vi "SCA-RT.vi"() -> ()   [LabVIEW 2016]
uses:
  Controls/SCA states.ctl
  Controls/Gate Valve Readback.ctl
  Controls/Vertical Rod states.ctl
  Controls/Horizontal Rod states.ctl
  Controls/GP307 cluster.ctl
  Controls/SCA commands.ctl
  Controls/SCA Bypass control.ctl
  Controls/Sample Changer Settings.ctl
  <vilib>/Platform/TimedLoop/XDataNode/timing_clust.ctl
  <vilib>/Platform/TimedLoop/XDataNode/nitl_modes.ctl
  <vilib>/Platform/TimedLoop/XDataNode/wakeup.ctl
  Controls/Encoder bit cluster.ctl
  Controls/Minimum Times.ctl
  <vilib>/Analysis/baseanly.llb/Mean (DBL).vi
  <vilib>/Instr/_visa.llb/VISA Configure Serial Port (Instr).vi
  <vilib>/Motion/Express/_s/nimc.fb.straightLineMove.startStraightLineMove.axis.modeRelative.0.vi
  <vilib>/Platform/TimedLoop/XDataNode/loadnilvce.vi
  <vilib>/Motion/BlockNode/FB.NIMotion.xnode
  <vilib>/Platform/TimedLoop/XDataNode/XDataNode.xnode
  <vilib>/Platform/TimedLoop/XDataNode/XDNodeRunTimeDep.lvlib
  <vilib>/Analysis/NI_AALBase.lvlib
  <vilib>/NI_Real-Time Target Support.lvlib
panel:
  out "Encoder Offset":i32
  out "SCA settings":T1
  out "Bypass error":errorcluster
  out "HV Readback error":errorcluster
  out "SCA command monitor error":errorcluster
  in  "Insert Rod Bypass":bool
  in  "Retract Rod Bypass":bool
  in  "Sample Rod Bypass":bool
  in  "Wheel GV Bypass":bool
  out "Bypass Control":T2
  out "Timeouts":T3
  out "Immersion Lens I set":dbl
  out "Immersion Lens V Set":dbl
  out "Settings Update error":errorcluster
  out "SCA Command":T4=enum."Retract insert rod"
  out "Encoder error":errorcluster
  out "Convectron readback error":errorcluster
  out "HV Control error":errorcluster
  out "Rotate Wheel error":errorcluster
  out "Ion Source Vac Cluster":T5
  out "Bellows Vac Cluster":T5
  out "SCA-cRIO error":errorcluster
  out "Rollover Sample":u16=54
  out "Insert Rod Status":T6
  out "Retract Rod Status":T6
  out "Sample Rod status":T7
  out "Wheel GV":T8
  out "Raw bits":bool[](array[boolean])
  out "Converted bits":bool[](array[boolean])
  out "Immersion Lens I read":dbl format="%0.2f"
  out "Immersion Lens V read":dbl format="%0.2f"
  out "SCA next state":T9
  out "Extractor I read":dbl
  out "Extractor V read":dbl
  out "Extractor V set":dbl
  out "Cathode V read":dbl
  out "Cathode I read":dbl
  out "Cathode V set":dbl
  out "New Move":dbl
  out "Encoder Destination":dbl
  out "Step Window Radius":u8=2
  out "In Range?":bool
  out "Window Limit 2":u32
  out "Window Limit 1":u32
  out "Encoder position":u16
  out "action":string
  out "Vac Readback error":errorcluster
  out "Sample Wheel Convectron":string
  out "Sample Rod UP sensor":bool
  out "Sample Rod DOWN sensor":bool
  out "Rotation done":bool
  out "Insert Rod IN sensor":bool
  out "Insert Rod OUT sensor":bool
  out "Retract Rod IN sensor":bool
  out "Retract Rod OUT sensor":bool
  out "Sensor error":errorcluster
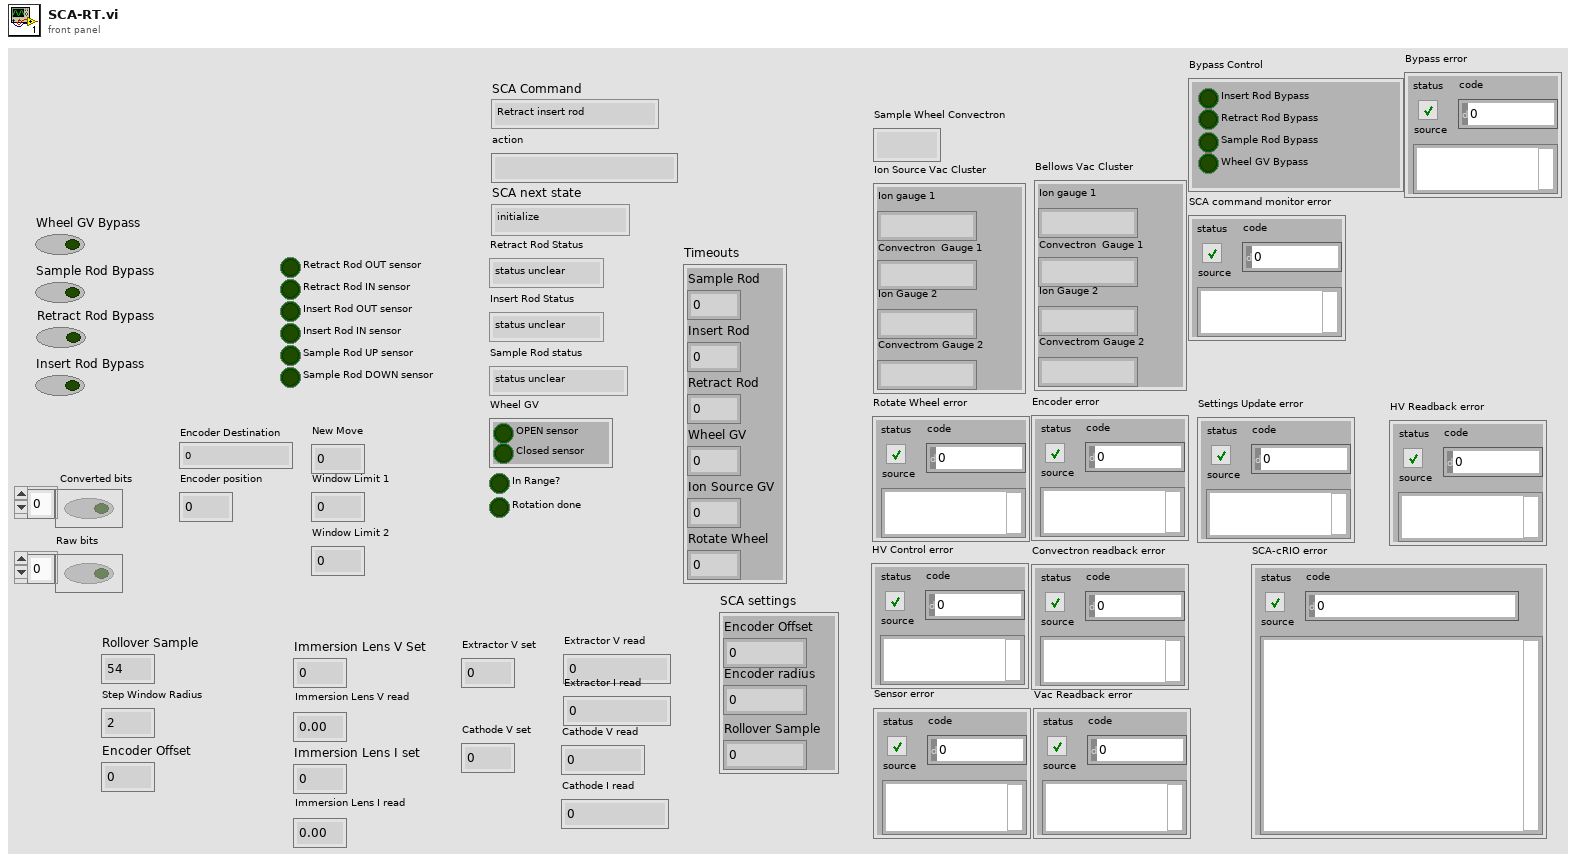
[diagram p1: front panel]
types:
  T1 = typedef "Sample Changer Settings.ctl" = cluster{"Encoder Offset":i32, "Encoder radius":u8, "Rollover Sample":u16}
  T2 = typedef "SCA Bypass control.ctl" = cluster{"Insert Rod Bypass":bool, "Retract Rod Bypass":bool, "Sample Rod Bypass":bool, "Wheel GV Bypass":bool}
  T3 = cluster{"Sample Rod":u16, "Insert Rod":u16, "Retract Rod":u16, "Wheel GV":u16, "Ion Source GV":u16, "Rotate Wheel":u16}
  T4 = typedef "SCA commands.ctl" = enum16{"Wait", "Shutdown", "Retract insert rod", "Insert insert rod", "Retract retract rod", "Insert retract rod", "Retract sample rod", "Insert sample rod", "Open wheel GV", "Close wheel GV", "Open ion source GV", "Close ion source GV", "Pump out source", "Vent source", "Rotate wheel randomly", "Rotate wheel", "Start random sample change", "Start sample change"}
  T5 = typedef "GP307 cluster.ctl" = cluster{"Ion gauge 1":string, "Convectron  Gauge 1 ":string, "Ion Gauge 2":string, "Convectrom Gauge 2":string}
  T6 = typedef "Horizontal Rod states.ctl" = enum16{"status unclear", "rod in", "rod out"}
  T7 = typedef "Vertical Rod states.ctl" = enum16{"status unclear", "rod down", "rod up"}
  T8 = typedef "Gate Valve Readback.ctl" = cluster{"OPEN sensor":bool, "Closed sensor":bool}
  T9 = typedef "SCA states.ctl" = enum16{"initialize", "wait", "change sample start", "change sample", "check position", "rotate wheel", "sample change complete", "sample rod up", "sample rod down", "retract rod in", "retract rod out", "insert rod in", "insert rod out", "wheel GV open", "wheel GV close", "vent source", "pump source", "shutdown"}
  T10 = cluster{"Sample Rod":u32, "Insert Rod":u32, "Retract Rod":u32, "Wheel GV":u32, "Ion Source GV":u32, "Rotate Wheel":u32}
  T11 = typedef "Minimum Times.ctl" = cluster{"Rotate Wheel Minimum Time":u32}
  T12 = typedef "XDNodeRunTimeDep.lvlib/timing_clust.ctl" = cluster{"Expected End [f-1]":u64, "Actual End [f-1]":u64, "Finished Late? [f-1]":bool, "Expected End [i-1]":u64, "Actual End [i-1]":u64, "Finished Late? [i-1]":bool, "Expected Start [i]":u64, "Actual Start [i]":u64, "Expected Start [f]":u64, "Actual Start [f]":u64, "Source Name":string, "Structure Name":string, "Period":i64, "Deadline":i64, "Offset":i64, "Start":i64, "Priority":i32, "Timeout":i32, "Mode":T13, "Wakeup Reason":T14, "Error":errorcluster, "Source Type":string, "Secondary Source Type":string, "Global End Time":u64, "Global Start Time":u64, "Frame Duration":u64, "Iteration Duration":u64, "Assigned CPU":i32, "I/O Scan Engine Mode":u32}
  T13 = typedef "XDNodeRunTimeDep.lvlib/nitl_modes.ctl" = enum32{"No Change", "Process missed periods, maintain original phase", "Discard missed periods, maintain original phase", "Process missed periods, ignore original phase", "Discard missed periods, ignore original phase"}
  T14 = typedef "XDNodeRunTimeDep.lvlib/wakeup.ctl" = enum32{"Normal", "Aborted", "Asynchronous wakeup", "Timing source error", "Timed loop error", "Timeout"}
  T15 = typedef "Encoder bit cluster.ctl" = cluster{"MSB":bool, "13th bit":bool, "12th bit":bool, "11th bit":bool, "10th bit":bool, "9th bit":bool, "8th bit":bool, "7th bit":bool, "6th bit":bool, "5th bit":bool, "4th bit":bool, "3rd bit":bool, "2nd bit":bool, "LSB":bool}
  T16 = typedef "GV states.ctl" = enum16{"status unclear", "closed", "open"}
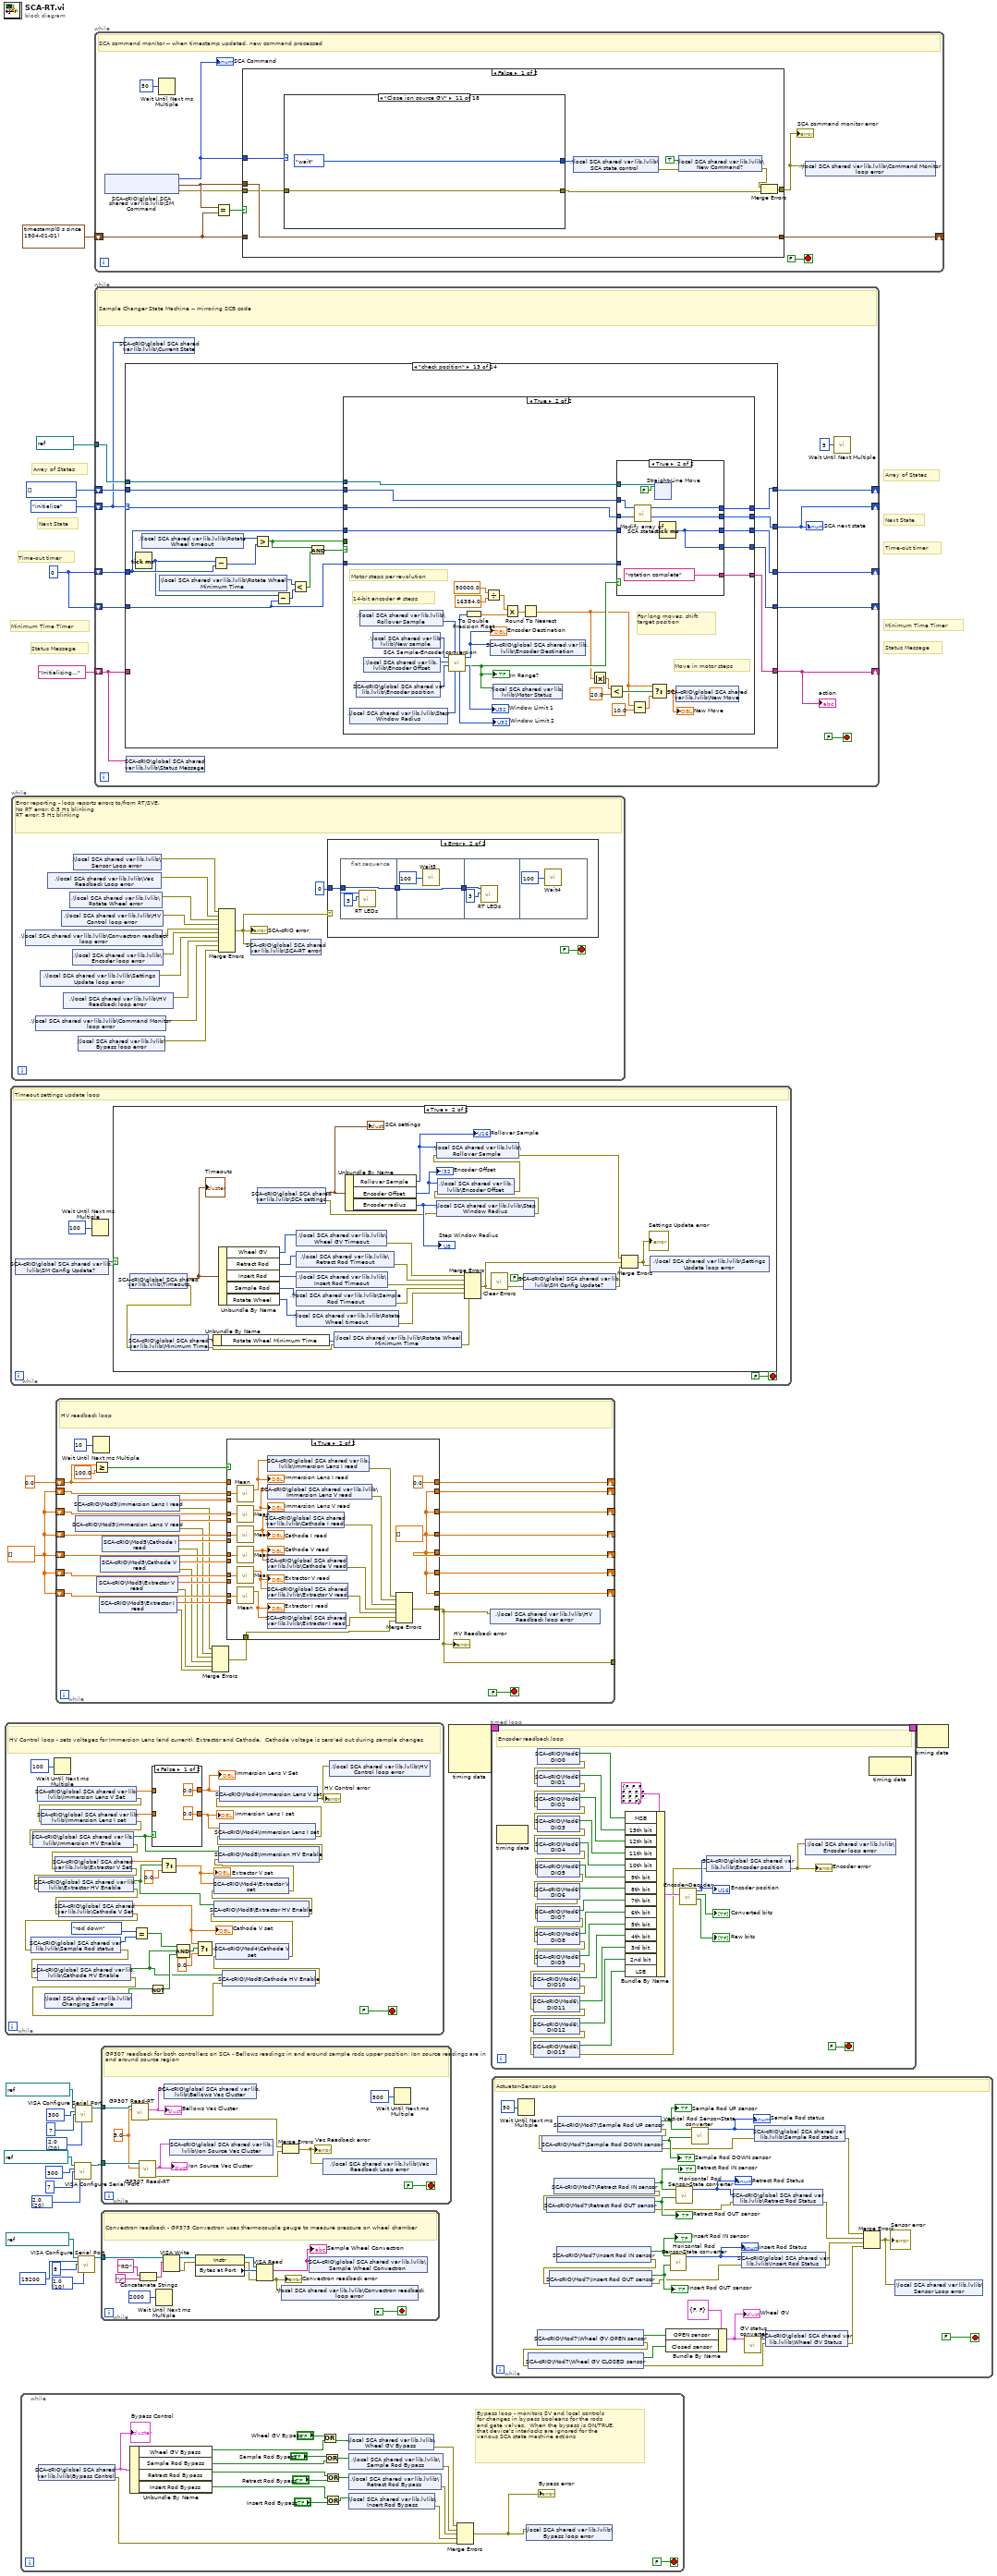
[diagram p0: block diagram]
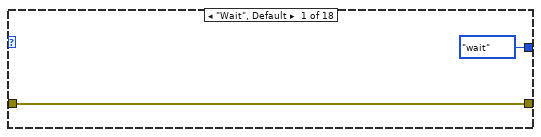
[diagram p2: hidden frame]
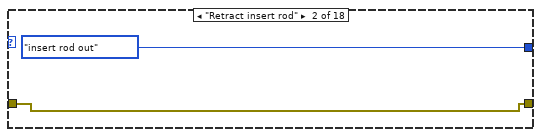
[diagram p3: hidden frame]
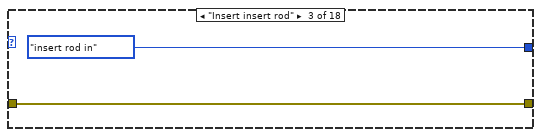
[diagram p4: hidden frame]
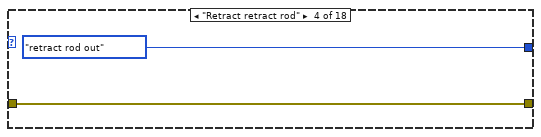
[diagram p5: hidden frame]
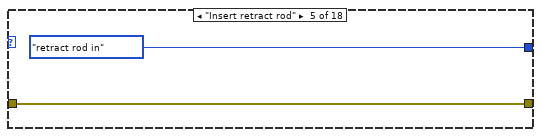
[diagram p6: hidden frame]
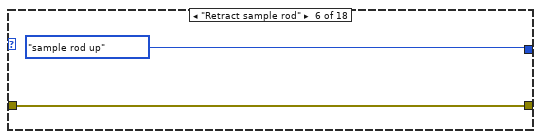
[diagram p7: hidden frame]
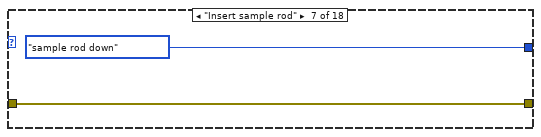
[diagram p8: hidden frame]
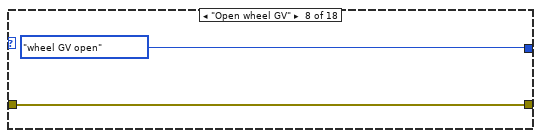
[diagram p9: hidden frame]
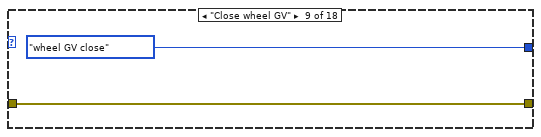
[diagram p10: hidden frame]
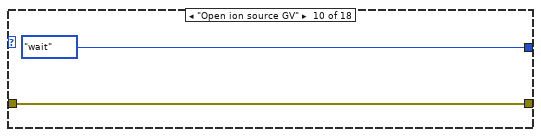
[diagram p11: hidden frame]
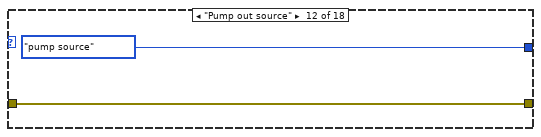
[diagram p12: hidden frame]
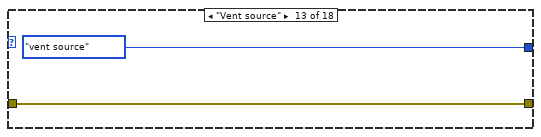
[diagram p13: hidden frame]
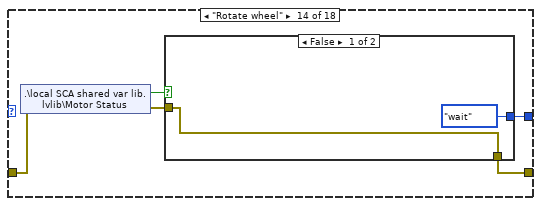
[diagram p14: hidden frame]
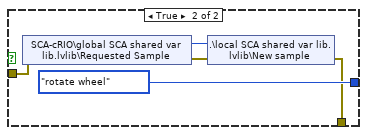
[diagram p15: hidden frame]
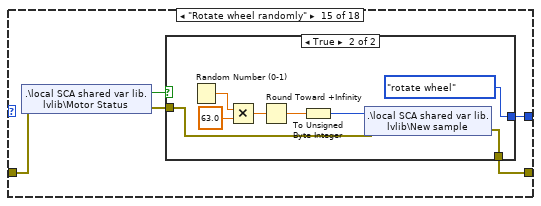
[diagram p16: hidden frame]
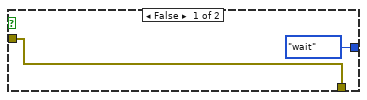
[diagram p17: hidden frame]
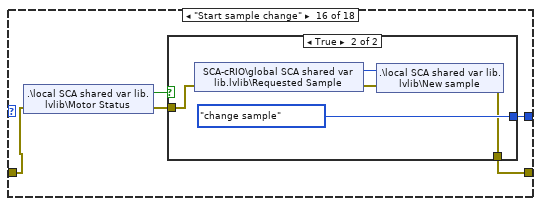
[diagram p18: hidden frame]
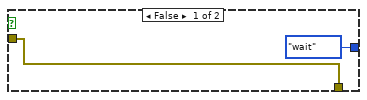
[diagram p19: hidden frame]
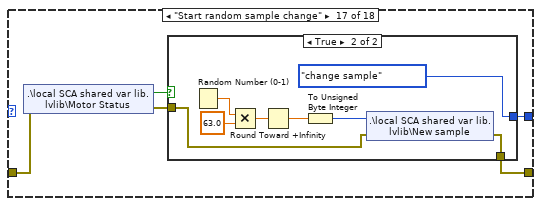
[diagram p20: hidden frame]
diagram:
  w3 = dbl[] []
  w20 = u16 20 items=["1.0"=10, "1.5"=15, "2.0"=20] ("stop bits (10: 1 bit)")
  w24 = u16 10 items=["1.0"=10, "1.5"=15, "2.0"=20] ("stop bits (10: 1 bit)")
  w14 = u16 20 items=["1.0"=10, "1.5"=15, "2.0"=20] ("stop bits (10: 1 bit)")
  w8 = u32 0
  w25 = T9[] [] items=["initialize", "wait", "change sample start", "change sample", "check position", "rotate wheel", "sample change complete", "sample rod up", "sample rod down", "retract rod in", "retract rod out", "insert rod in", "insert rod out", "wheel GV open", "wheel GV close", "vent source", "pump source", "shutdown"]
  # "Status Message"
  # "Array of States"
  # "Next State"
  # "Time-out timer"
  # "Minimum Time Timer"
  # "Status Message"
  # "Array of States"
  # "Next State"
  # "Time-out timer"
  # "Minimum Time Timer"
  n1 = while {
    stop <- FALSE stop-if-true
    # "HV Control loop - sets voltages for Immersion Lens (and current), Extractor and Cathode.  Cathode voltage is zero'ed out during sample changes"
    n2 = shared-variable "SCA-cRIO\\global SCA shared var lib.lvlib\\Immersion Lens V Set"() -> (w47:dbl, error out=w54:errorcluster)  [unwired: 1 in]
    n3 = shared-variable "SCA-cRIO\\global SCA shared var lib.lvlib\\Immersion Lens I set"(error in=w54) -> (w45:dbl, error out=w43:errorcluster)
    n4 = shared-variable "SCA-cRIO\\global SCA shared var lib.lvlib\\Immersion HV Enable"(error in=w43) -> (w27:bool, error out=w42:errorcluster)
    n5 = shared-variable ".\\local SCA shared var lib.lvlib\\Changing Sample"() -> (w59:bool)  [unwired: 1 in, 1 out]
    n6 = Wait Until Next ms Multiple(millisecond multiple=u32 100) -> ()  [unwired: 1 out]
    n7 = shared-variable "SCA-cRIO\\global SCA shared var lib.lvlib\\Extractor V Set"(error in=w42) -> (w40:dbl, error out=w41:errorcluster)
    n8 = shared-variable "SCA-cRIO\\global SCA shared var lib.lvlib\\Extractor HV Enable"(error in=w41) -> (w26:bool, error out=w37:errorcluster)
    n9 = shared-variable "SCA-cRIO\\global SCA shared var lib.lvlib\\Cathode V Set"(error in=w37) -> (w57:dbl, error out=w53:errorcluster)
    "Cathode V set" <- w57
    n10 = shared-variable "SCA-cRIO\\global SCA shared var lib.lvlib\\Sample Rod status"(error in=w53) -> (w49:T7, error out=w35:errorcluster)
    n11 = shared-variable "SCA-cRIO\\global SCA shared var lib.lvlib\\Cathode HV Enable"(error in=w35) -> (w34:bool, error out=w33:errorcluster)
    n12 = Equal?(x=Vertical_Rod_states."rod down", y=w49) -> (x = y?=w50:bool)
    n13 = Not(x=w59) -> (.not. x?=w36:bool)
    n14 = case shown="False" w27 {
      tunnel: [0.0 ("Double") w65] -> w46
      tunnel: w47 -> [_ w65]
      tunnel: w45 -> [_ w64]
      tunnel: [0.0 ("Double") w64] -> w44
      frame False {
      }
      frame True {
      }
    }
    "Immersion Lens V Set" <- w46
    "Immersion Lens I set" <- w44
    n15 = Select(t=w40, s=w26, f=0.0) -> (s? t:f=w39:dbl)
    "Extractor V set" <- w39
    n16 = Compound Arithmetic op=AND(w50, w34, w36) -> (w58:bool)
    n17 = Select(t=w57, s=w58, f=0.0) -> (s? t:f=w55:dbl)
    n18 = shared-variable "SCA-cRIO\\Mod8\\Cathode HV Enable"(w34, error in=w33) -> (error out=w32:errorcluster)
    n19 = shared-variable "SCA-cRIO\\Mod4\\Cathode V set"(w55, error in=w32) -> (error out=w31:errorcluster)
    n20 = shared-variable "SCA-cRIO\\Mod8\\Extractor HV Enable"(w26, error in=w31) -> (error out=w30:errorcluster)
    n21 = shared-variable "SCA-cRIO\\Mod4\\Extractor V set"(w39, error in=w30) -> (error out=w28:errorcluster)
    n22 = shared-variable "SCA-cRIO\\Mod8\\Immersion HV Enable"(w27, error in=w28) -> (error out=w29:errorcluster)
    n23 = shared-variable "SCA-cRIO\\Mod4\\Immersion Lens I set"(w44, error in=w29) -> (error out=w52:errorcluster)
    n24 = shared-variable "SCA-cRIO\\Mod4\\Immersion Lens V set"(w46, error in=w52) -> (error out=w51:errorcluster)
    "HV Control error" <- w51
    n25 = shared-variable ".\\local SCA shared var lib.lvlib\\HV Control loop error"(w51) -> ()  [unwired: 1 in, 1 out]
  }
  n26 = while {
    stop <- FALSE stop-if-true
    # "Timeout settings update loop"
    n27 = shared-variable "SCA-cRIO\\global SCA shared var lib.lvlib\\SM Config Update?"() -> (w68:bool)  [unwired: 1 in, 1 out]
    n28 = Wait Until Next ms Multiple(millisecond multiple=u32 100) -> ()  [unwired: 1 out]
    n29 = case shown="True" w68 {
      frame False {
      }
      frame True {
        n30 = shared-variable "SCA-cRIO\\global SCA shared var lib.lvlib\\Timeouts"() -> (w96:T10, error out=w79:errorcluster)  [unwired: 1 in]
        "Timeouts" <- w96
        n31 = shared-variable "SCA-cRIO\\global SCA shared var lib.lvlib\\Minimum Time"(error in=w79) -> (w81:T11, error out=w78:errorcluster)
        n32 = Unbundle By Name(w81) -> ("Rotate Wheel Minimum Time"=w80:u32)
        n33 = Unbundle By Name(w96) -> ("Wheel GV"=w95:u32, "Retract Rod"=w82:u32, "Insert Rod"=w89:u32, "Sample Rod"=w86:u32, "Rotate Wheel"=w85:u32)
        n34 = shared-variable "SCA-cRIO\\global SCA shared var lib.lvlib\\SCA settings"() -> (w76:T1, error out=w73:errorcluster)  [unwired: 1 in]
        "SCA settings" <- w76
        n35 = shared-variable ".\\local SCA shared var lib.lvlib\\Wheel GV Timeout"(w95) -> (error out=w94:errorcluster)  [unwired: 1 in]
        n36 = shared-variable ".\\local SCA shared var lib.lvlib\\Retract Rod Timeout"(w82) -> (error out=w88:errorcluster)  [unwired: 1 in]
        n37 = shared-variable ".\\local SCA shared var lib.lvlib\\Insert Rod Timeout"(w89) -> (error out=w87:errorcluster)  [unwired: 1 in]
        n38 = shared-variable ".\\local SCA shared var lib.lvlib\\Sample Rod Timeout"(w86) -> (error out=w84:errorcluster)  [unwired: 1 in]
        n39 = shared-variable ".\\local SCA shared var lib.lvlib\\Rotate Wheel timeout"(w85) -> (error out=w83:errorcluster)  [unwired: 1 in]
        n40 = shared-variable ".\\local SCA shared var lib.lvlib\\Rotate Wheel Minimum Time"(w80, error in=w78) -> (error out=w77:errorcluster)
        n41 = Unbundle By Name(w76) -> ("Rollover Sample"=w71:u16, "Encoder Offset"=w74:i32, "Encoder radius"=w75:u8)
        "Step Window Radius" <- w75
        "Rollover Sample" <- w71
        "Encoder Offset" <- w74
        n42 = shared-variable ".\\local SCA shared var lib.lvlib\\Step Window Radius"(w75, error in=w73) -> (error out=w72:errorcluster)
        n43 = shared-variable ".\\local SCA shared var lib.lvlib\\Encoder Offset"(w74, error in=w72) -> (error out=w70:errorcluster)
        n44 = shared-variable ".\\local SCA shared var lib.lvlib\\Rollover Sample"(w71, error in=w70) -> (error out=w69:errorcluster)
        n45 = Merge Errors(w94, w88, w87, w84, w83, w77) -> (w92:errorcluster)
        n46 = call <vilib>:"Clear Errors.vi"("error in (no error)"=w92) -> ("error out"=w93:errorcluster)  [unwired: 5 in, 1 out]
        n47 = shared-variable "SCA-cRIO\\global SCA shared var lib.lvlib\\SM Config Update?"(FALSE ("SM Config Update?"), error in=w93) -> (error out=w91:errorcluster)
        n48 = Merge Errors(w69, w92, w91) -> (w90:errorcluster)
        "Settings Update error" <- w90
        n49 = shared-variable ".\\local SCA shared var lib.lvlib\\Settings Update loop error"(w90) -> ()  [unwired: 1 in, 1 out]
      }
    }
  }
  n50 = while {
    stop <- FALSE stop-if-true
    # "Error reporting - loop reports errors to/from RT/SVE. \nNo RT error: 0.5 Hz blinking\nRT error: 5 Hz blinking"
    n51 = shared-variable ".\\local SCA shared var lib.lvlib\\Convectron readback loop error"() -> (w103:errorcluster)  [unwired: 1 in, 1 out]
    n52 = shared-variable ".\\local SCA shared var lib.lvlib\\Command Monitor loop error"() -> (w99:errorcluster)  [unwired: 1 in, 1 out]
    n53 = shared-variable ".\\local SCA shared var lib.lvlib\\Settings Update loop error"() -> (w101:errorcluster)  [unwired: 1 in, 1 out]
    n54 = shared-variable ".\\local SCA shared var lib.lvlib\\Vac Readback Loop error"() -> (w108:errorcluster)  [unwired: 1 in, 1 out]
    n55 = shared-variable ".\\local SCA shared var lib.lvlib\\HV Control loop error"() -> (w104:errorcluster)  [unwired: 1 in, 1 out]
    n56 = shared-variable ".\\local SCA shared var lib.lvlib\\HV Readback loop error"() -> (w100:errorcluster)  [unwired: 1 in, 1 out]
    n57 = shared-variable ".\\local SCA shared var lib.lvlib\\Rotate Wheel error"() -> (w105:errorcluster)  [unwired: 1 in, 1 out]
    n58 = shared-variable ".\\local SCA shared var lib.lvlib\\Encoder loop error"() -> (w102:errorcluster)  [unwired: 1 in, 1 out]
    n59 = shared-variable ".\\local SCA shared var lib.lvlib\\Sensor Loop error"() -> (w109:errorcluster)  [unwired: 1 in, 1 out]
    n60 = shared-variable ".\\local SCA shared var lib.lvlib\\Bypass loop error"() -> (w98:errorcluster)  [unwired: 1 in, 1 out]
    n61 = Merge Errors(w109, w108, w105, w104, w103, w102, w101, w100, w99, w98) -> (w107:errorcluster)
    "SCA-cRIO error" <- w107
    n62 = shared-variable "SCA-cRIO\\global SCA shared var lib.lvlib\\SCA-RT error"(w107) -> ()  [unwired: 1 in, 1 out]
    n63 = case shown="Error" w107 {
      tunnel: 0 -> [w113 w121]
      frame No Error {
        n64 = flat-sequence {
          tunnel: w113 -> [w114]
          tunnel: [w114] -> w111
          tunnel: [w116] -> w112
          tunnel: w111 -> [w116]
          tunnel: w112 -> [w118]
          frame #0 {
            n65 = call <vilib>:"RT LEDs.vi"("State"=3, "LED Num"=w114) -> ()  [unwired: 4 in, 2 out]
          }
          frame #1 {
            n66 = call "Wait"("Count(mSec)"=u16 1000) -> ()  [unwired: 1 out]
          }
          frame #2 {
            n67 = call <vilib>:"RT LEDs.vi"("State"=3, "LED Num"=w118) -> ()  [unwired: 4 in, 2 out]
          }
          frame #3 {
            n68 = call "Wait2"("Count(mSec)"=u16 1000) -> ()  [unwired: 1 out]
          }
        }
      }
      frame Error {
        n69 = flat-sequence {
          tunnel: [w124] -> w123
          tunnel: w121 -> [w124]
          tunnel: w123 -> [w126]
          tunnel: [w126] -> w122
          tunnel: w122 -> [w128]
          frame #0 {
            n70 = call <vilib>:"RT LEDs.vi"("State"=3, "LED Num"=w124) -> ()  [unwired: 4 in, 2 out]
          }
          frame #1 {
            n71 = call "Wait3"("Count(mSec)"=u16 100) -> ()  [unwired: 1 out]
          }
          frame #2 {
            n72 = call <vilib>:"RT LEDs.vi"("State"=3, "LED Num"=w128) -> ()  [unwired: 4 in, 2 out]
          }
          frame #3 {
            n73 = call "Wait4"("Count(mSec)"=u16 100) -> ()  [unwired: 1 out]
          }
        }
      }
    }
  }
  n74 = while {
    stop <- FALSE stop-if-true
    # "Bypass loop - monitors SV and local controls\nfor changes in bypass booleans for the rods \nand gate valves.  When the bypass is ON/TRUE,\nthat device's interlocks are ignored for the \nvarious SCA state machine actions"
    n75 = shared-variable "SCA-cRIO\\global SCA shared var lib.lvlib\\Bypass Control"() -> (w144:T2, error out=w132:errorcluster)  [unwired: 1 in]
    "Bypass Control" <- w144
    n76 = Unbundle By Name(w144) -> ("Wheel GV Bypass"=w141:bool, "Sample Rod Bypass"=w140:bool, "Retract Rod Bypass"=w139:bool, "Insert Rod Bypass"=w138:bool)
    n77 = Or(x="Wheel GV Bypass", y=w141) -> (x .or. y?=w148:bool)
    n78 = Or(x="Sample Rod Bypass", y=w140) -> (x .or. y?=w147:bool)
    n79 = Or(x=w139, y="Retract Rod Bypass") -> (x .or. y?=w145:bool)
    n80 = Or(x=w138, y="Insert Rod Bypass") -> (x .or. y?=w146:bool)
    n81 = shared-variable ".\\local SCA shared var lib.lvlib\\Wheel GV Bypass"(w148) -> (error out=w136:errorcluster)  [unwired: 1 in]
    n82 = shared-variable ".\\local SCA shared var lib.lvlib\\Sample Rod Bypass"(w147) -> (error out=w135:errorcluster)  [unwired: 1 in]
    n83 = shared-variable ".\\local SCA shared var lib.lvlib\\Retract Rod Bypass"(w145) -> (error out=w134:errorcluster)  [unwired: 1 in]
    n84 = shared-variable ".\\local SCA shared var lib.lvlib\\Insert Rod Bypass"(w146) -> (error out=w133:errorcluster)  [unwired: 1 in]
    n85 = Merge Errors(w136, w135, w134, w133, w132) -> (w131:errorcluster)
    "Bypass error" <- w131
    n86 = shared-variable ".\\local SCA shared var lib.lvlib\\Bypass loop error"(w131) -> ()  [unwired: 1 in, 1 out]
  }
  n87 = while {
    shift-right: [w175] -> _
    shift-left: 0.0 ("AI1") -> [w178]
    shift-right: [w173] -> _
    shift-left: w3 -> [w172]
    shift-right: [w174] -> _
    shift-left: w3 -> [w171]
    shift-right: [w169] -> _
    shift-left: w3 -> [w168]
    shift-right: [w166] -> _
    shift-left: w3 -> [w165]
    shift-right: [w160] -> _
    shift-left: w3 -> [w163]
    shift-right: [w159] -> _
    shift-left: w3 -> [w164]
    tunnel: [w151] -> _
    stop <- FALSE stop-if-true
    # "HV readback loop"
    n88 = shared-variable "SCA-cRIO\\Mod5\\Immersion Lens V read"() -> (w161:dbl, error out=w157:errorcluster)  [unwired: 1 in]
    n89 = shared-variable "SCA-cRIO\\Mod5\\Immersion Lens I read"() -> (w162:dbl, error out=w158:errorcluster)  [unwired: 1 in]
    n90 = Wait Until Next ms Multiple(millisecond multiple=u32 10) -> ()  [unwired: 1 out]
    n91 = Greater Or Equal?(x=w178, y=100.0) -> (x >= y?=w176:bool)
    n92 = shared-variable "SCA-cRIO\\Mod5\\Extractor V read"() -> (w170:dbl, error out=w154:errorcluster)  [unwired: 1 in]
    n93 = shared-variable "SCA-cRIO\\Mod5\\Extractor I read"() -> (w167:dbl, error out=w153:errorcluster)  [unwired: 1 in]
    n94 = shared-variable "SCA-cRIO\\Mod5\\Cathode V read"() -> (w180:dbl, error out=w155:errorcluster)  [unwired: 1 in]
    n95 = shared-variable "SCA-cRIO\\Mod5\\Cathode I read"() -> (w179:dbl, error out=w156:errorcluster)  [unwired: 1 in]
    n96 = Merge Errors(w158, w157, w156, w155, w154, w153) -> (w152:errorcluster)
    n97 = case shown="True" w176 {
      tunnel: w180 -> [w199 _]
      tunnel: w179 -> [w200 _]
      tunnel: w178 -> [w203 _]
      tunnel: [w202 0.0 ("AI1")] -> w175
      tunnel: [w201 w215] -> w174
      tunnel: [w198 w215] -> w173
      tunnel: w172 -> [w197 w223]
      tunnel: w171 -> [w196 w224]
      tunnel: w170 -> [w195 _]
      tunnel: [w194 w215] -> w169
      tunnel: w168 -> [w193 w222]
      tunnel: w167 -> [w192 _]
      tunnel: [w191 w215] -> w166
      tunnel: w165 -> [w190 w221]
      tunnel: w164 -> [w189 w214]
      tunnel: w163 -> [w188 w213]
      tunnel: w162 -> [w187 _]
      tunnel: w161 -> [w186 _]
      tunnel: [w185 w215] -> w160
      tunnel: [w184 w215] -> w159
      tunnel: w152 -> [w183 w210]
      tunnel: [w183 w204] -> w151
      frame False {
        n98 = Build Array (concatenate)(w187, w188) -> (w185:dbl[])
        n99 = Build Array (concatenate)(w186, w189) -> (w184:dbl[])
        n100 = Build Array (concatenate)(w200, w196) -> (w201:dbl[])
        n101 = Build Array (concatenate)(w199, w197) -> (w198:dbl[])
        n102 = Build Array (concatenate)(w195, w193) -> (w194:dbl[])
        n103 = Build Array (concatenate)(w192, w190) -> (w191:dbl[])
        n104 = Increment(x=w203) -> (x+1=w202:dbl)
      }
      frame True {
        w215 = dbl[] []
        n105 = call-poly <vilib>:"Mean.vi"("X"=w213) -> ("mean"=w212:dbl)  [unwired: 1 out]
        "Immersion Lens I read" <- w212
        n106 = call-poly <vilib>:"Mean.vi"("X"=w214) -> ("mean"=w216:dbl)  [unwired: 1 out]
        "Immersion Lens V read" <- w216
        n107 = call-poly <vilib>:"Mean.vi"("X"=w224) -> ("mean"=w220:dbl)  [unwired: 1 out]
        "Cathode I read" <- w220
        n108 = call-poly <vilib>:"Mean.vi"("X"=w223) -> ("mean"=w219:dbl)  [unwired: 1 out]
        "Cathode V read" <- w219
        n109 = call-poly <vilib>:"Mean.vi"("X"=w222) -> ("mean"=w218:dbl)  [unwired: 1 out]
        "Extractor V read" <- w218
        n110 = call-poly <vilib>:"Mean.vi"("X"=w221) -> ("mean"=w217:dbl)  [unwired: 1 out]
        "Extractor I read" <- w217
        n111 = shared-variable "SCA-cRIO\\global SCA shared var lib.lvlib\\Immersion Lens I read"(w212) -> (error out=w211:errorcluster)  [unwired: 1 in]
        n112 = shared-variable "SCA-cRIO\\global SCA shared var lib.lvlib\\Immersion Lens V read"(w216) -> (error out=w209:errorcluster)  [unwired: 1 in]
        n113 = shared-variable "SCA-cRIO\\global SCA shared var lib.lvlib\\Cathode I read"(w220) -> (error out=w208:errorcluster)  [unwired: 1 in]
        n114 = shared-variable "SCA-cRIO\\global SCA shared var lib.lvlib\\Cathode V read"(w219) -> (error out=w207:errorcluster)  [unwired: 1 in]
        n115 = shared-variable "SCA-cRIO\\global SCA shared var lib.lvlib\\Extractor V read"(w218) -> (error out=w206:errorcluster)  [unwired: 1 in]
        n116 = shared-variable "SCA-cRIO\\global SCA shared var lib.lvlib\\Extractor I read"(w217) -> (error out=w205:errorcluster)  [unwired: 1 in]
        n117 = Merge Errors(w211, w209, w208, w207, w206, w205, w210) -> (w204:errorcluster)
      }
    }
    "HV Readback error" <- w151
    n118 = shared-variable ".\\local SCA shared var lib.lvlib\\HV Readback loop error"(w151) -> ()  [unwired: 1 in, 1 out]
  }
  n119 = call-poly "VISA Configure Serial Port"("VISA resource name"=refnum<visa-resource-name> "ASRL6::INSTR", "baud rate (9600)"=u32 300, "data bits (8)"=u16 7, "stop bits (10: 1 bit)"=w14) -> ("VISA resource name out"=w15:refnum<visa-resource-name>)  [unwired: 10 in, 1 out]
  n120 = call-poly "VISA Configure Serial Port"("VISA resource name"=refnum<visa-resource-name> "ASRL8::INSTR", "baud rate (9600)"=u32 300, "data bits (8)"=u16 7, "stop bits (10: 1 bit)"=w20) -> ("VISA resource name out"=w21:refnum<visa-resource-name>)  [unwired: 10 in, 1 out]
  n121 = call-poly "VISA Configure Serial Port"("VISA resource name"=refnum<visa-resource-name> "ASRL7::INSTR", "baud rate (9600)"=u32 19200, "data bits (8)"=u16 8, "stop bits (10: 1 bit)"=w24) -> ("VISA resource name out"=w10:refnum<visa-resource-name>)  [unwired: 10 in, 1 out]
  n122 = while {
    shift-right: [w226] -> _
    shift-left: SCA_states."initialize" ("SC2 state") -> [w227]
    shift-right: [w230] -> _
    shift-left: w25 -> [w236]
    shift-right: [w234] -> _
    shift-left: w8 -> [w235]
    shift-right: [w228] -> _
    shift-left: "Initializing..." -> [w231]
    shift-right: [w232] -> _
    shift-left: w8 -> [w233]
    tunnel: refnum<k21> "Axis 1" ("resource") -> [w237]
    stop <- FALSE ("stop 2") stop-if-true
    # "Sample Changer State Machine -- mirroring SCB code"
    n123 = shared-variable "SCA-cRIO\\global SCA shared var lib.lvlib\\Current State"(w227) -> ()  [unwired: 1 in, 1 out]
    n124 = case shown="\"check position\"" w227 {
      selector: w227 -> [_ _ w277 w310 w374 w402 w471 w537 w565 w638 w661 _ w723 w838]
      tunnel: w237 -> [_ _ _ _ _ _ _ _ _ _ _ w685 w719 _]
      tunnel: [SCA_states."wait" ("SC2 state") w256 w282 w306 w369 w397 w466 w532 w560 w634 w660 w677 w720 w836] -> w226
      tunnel: w236 -> [w247 _ w279 w312 w375 w403 w472 w538 w566 w639 w663 w678 w718 w839]
      tunnel: w235 -> [w250 _ w278 w308 w372 w399 w469 w535 w562 w636 _ w667 w715 _]
      tunnel: [w250 w255 w278 w308 w372 w399 w469 w535 w562 w636 w664 w667 w721 w842] -> w234
      tunnel: [w247 w257 w281 w305 w368 w396 w465 w531 w561 w633 w662 w678 w717 w837] -> w230
      tunnel: w231 -> [w248 w253 _ _ _ _ _ _ _ _ w659 _ _ w835]
      tunnel: [w248 w253 w283 w309 w371 w400 w468 w534 w563 w632 w659 "done rotating, checking position" ("t") w716 w835] -> w228
      tunnel: w233 -> [w251 _ w284 w311 w373 w401 w470 w536 w564 w637 _ w680 w712 _]
      tunnel: [w251 w255 w280 w307 w370 w398 w467 w533 w559 w635 w664 w680 w722 w842] -> w232
      frame "initialize" {
        n125 = shared-variable ".\\local SCA shared var lib.lvlib\\Motor Status"(TRUE ("Motor Status")) -> ()  [unwired: 1 in, 1 out]
        n126 = shared-variable ".\\local SCA shared var lib.lvlib\\Changing Sample"(FALSE ("Changing Sample")) -> ()  [unwired: 1 in, 1 out]
        n127 = shared-variable "SCA-cRIO\\global SCA shared var lib - old.lvlib\\Start Sample Change"(FALSE ("start sample change")) -> ()  [unwired: 1 in, 1 out]
        n128 = shared-variable ".\\local SCA shared var lib.lvlib\\Rotate Wheel Minimum Time"(u16 1000 ("Rotate Wheel Minimum Time")) -> ()  [unwired: 1 in, 1 out]
        n129 = shared-variable ".\\local SCA shared var lib.lvlib\\Retract Rod Timeout"(u32 10000 ("Retract Rod Timeout")) -> ()  [unwired: 1 in, 1 out]
        n130 = shared-variable ".\\local SCA shared var lib.lvlib\\Wheel GV Timeout"(10000 ("Wheel GV Timeout")) -> ()  [unwired: 1 in, 1 out]
        n131 = shared-variable ".\\local SCA shared var lib.lvlib\\Rotate Wheel timeout"(u32 30000 ("Rotate Wheel timeout")) -> ()  [unwired: 1 in, 1 out]
        n132 = shared-variable ".\\local SCA shared var lib.lvlib\\Sample Rod Timeout"(u32 10000 ("Sample Rod Timeout")) -> ()  [unwired: 1 in, 1 out]
        n133 = shared-variable ".\\local SCA shared var lib.lvlib\\Insert Rod Timeout"(u32 10000 ("Insert Rod Timeout")) -> ()  [unwired: 1 in, 1 out]
      }
      frame "wait", Default {
        n134 = shared-variable ".\\local SCA shared var lib.lvlib\\New Command?"() -> (w254:bool)  [unwired: 1 in, 1 out]
        n135 = case shown="True" w254 {
          tunnel: [w259 w262] -> w257
          frame False {
            w259 = T9[] [enum."wait"] items=["initialize", "wait", "change sample start", "change sample", "check position", "rotate wheel", "sample change complete", "sample rod up", "sample rod down", "retract rod in", "retract rod out", "insert rod in", "insert rod out", "wheel GV open", "wheel GV close", "vent source", "pump source", "shutdown"]
          }
          frame True {
            n136 = shared-variable ".\\local SCA shared var lib.lvlib\\SCA state control"() -> (w261:T9)  [unwired: 1 in, 1 out]
            n137 = case shown="\"shutdown\"" w261 {
              tunnel: [w263 w264 w265 w266 w267 w268 w269 w270 w271 w272 w273 w274 w275 w276] -> w262
              frame "wheel GV close" {
                w263 = T9[] [enum."wheel GV close", enum."wait"] items=["initialize", "wait", "change sample start", "change sample", "check position", "rotate wheel", "sample change complete", "sample rod up", "sample rod down", "retract rod in", "retract rod out", "insert rod in", "insert rod out", "wheel GV open", "wheel GV close", "vent source", "pump source", "shutdown"]
              }
              frame "wheel GV open" {
                w264 = T9[] [enum."wheel GV open", enum."wait"] items=["initialize", "wait", "change sample start", "change sample", "check position", "rotate wheel", "sample change complete", "sample rod up", "sample rod down", "retract rod in", "retract rod out", "insert rod in", "insert rod out", "wheel GV open", "wheel GV close", "vent source", "pump source", "shutdown"]
              }
              frame "sample rod up" {
                w265 = T9[] [enum."sample rod up", enum."wait"] items=["initialize", "wait", "change sample start", "change sample", "check position", "rotate wheel", "sample change complete", "sample rod up", "sample rod down", "retract rod in", "retract rod out", "insert rod in", "insert rod out", "wheel GV open", "wheel GV close", "vent source", "pump source", "shutdown"]
              }
              frame "sample rod down" {
                w266 = T9[] [enum."sample rod down", enum."wait"] items=["initialize", "wait", "change sample start", "change sample", "check position", "rotate wheel", "sample change complete", "sample rod up", "sample rod down", "retract rod in", "retract rod out", "insert rod in", "insert rod out", "wheel GV open", "wheel GV close", "vent source", "pump source", "shutdown"]
              }
              frame "retract rod in" {
                w267 = T9[] [enum."retract rod in", enum."wait"] items=["initialize", "wait", "change sample start", "change sample", "check position", "rotate wheel", "sample change complete", "sample rod up", "sample rod down", "retract rod in", "retract rod out", "insert rod in", "insert rod out", "wheel GV open", "wheel GV close", "vent source", "pump source", "shutdown"]
              }
              frame "retract rod out" {
                w268 = T9[] [enum."retract rod out", enum."wait"] items=["initialize", "wait", "change sample start", "change sample", "check position", "rotate wheel", "sample change complete", "sample rod up", "sample rod down", "retract rod in", "retract rod out", "insert rod in", "insert rod out", "wheel GV open", "wheel GV close", "vent source", "pump source", "shutdown"]
              }
              frame "insert rod in" {
                w269 = T9[] [enum."insert rod in", enum."wait"] items=["initialize", "wait", "change sample start", "change sample", "check position", "rotate wheel", "sample change complete", "sample rod up", "sample rod down", "retract rod in", "retract rod out", "insert rod in", "insert rod out", "wheel GV open", "wheel GV close", "vent source", "pump source", "shutdown"]
              }
              frame "insert rod out" {
                w270 = T9[] [enum."insert rod out", enum."wait"] items=["initialize", "wait", "change sample start", "change sample", "check position", "rotate wheel", "sample change complete", "sample rod up", "sample rod down", "retract rod in", "retract rod out", "insert rod in", "insert rod out", "wheel GV open", "wheel GV close", "vent source", "pump source", "shutdown"]
              }
              frame "rotate wheel" {
                w271 = T9[] [enum."retract rod out", enum."insert rod out", enum."check position", enum."wait"] items=["initialize", "wait", "change sample start", "change sample", "check position", "rotate wheel", "sample change complete", "sample rod up", "sample rod down", "retract rod in", "retract rod out", "insert rod in", "insert rod out", "wheel GV open", "wheel GV close", "vent source", "pump source", "shutdown"]
              }
              frame "change sample" {
                w272 = T9[] [enum."change sample start", enum."sample rod up", enum."retract rod in", enum."retract rod out", enum."check position", enum."insert rod in", enum."insert rod out", enum."sample rod down", enum."sample change complete", enum."wait"] items=["initialize", "wait", "change sample start", "change sample", "check position", "rotate wheel", "sample change complete", "sample rod up", "sample rod down", "retract rod in", "retract rod out", "insert rod in", "insert rod out", "wheel GV open", "wheel GV close", "vent source", "pump source", "shutdown"]
              }
              frame "vent source" {
                w273 = T9[] [enum."sample rod up", enum."retract rod in", enum."retract rod out", enum."insert rod out", enum."wheel GV close", enum."wait"] items=["initialize", "wait", "change sample start", "change sample", "check position", "rotate wheel", "sample change complete", "sample rod up", "sample rod down", "retract rod in", "retract rod out", "insert rod in", "insert rod out", "wheel GV open", "wheel GV close", "vent source", "pump source", "shutdown"]
              }
              frame "pump source" {
                w274 = T9[] [enum."wheel GV open", enum."sample rod up", enum."check position", enum."insert rod in", enum."insert rod out", enum."sample rod down", enum."wait"] items=["initialize", "wait", "change sample start", "change sample", "check position", "rotate wheel", "sample change complete", "sample rod up", "sample rod down", "retract rod in", "retract rod out", "insert rod in", "insert rod out", "wheel GV open", "wheel GV close", "vent source", "pump source", "shutdown"]
              }
              frame "wait", Default {
                w275 = T9[] [enum."wait"] items=["initialize", "wait", "change sample start", "change sample", "check position", "rotate wheel", "sample change complete", "sample rod up", "sample rod down", "retract rod in", "retract rod out", "insert rod in", "insert rod out", "wheel GV open", "wheel GV close", "vent source", "pump source", "shutdown"]
              }
              frame "shutdown" {
                w276 = T9[] [enum."sample rod up", enum."retract rod in", enum."retract rod out", enum."wheel GV close", enum."wait"] items=["initialize", "wait", "change sample start", "change sample", "check position", "rotate wheel", "sample change complete", "sample rod up", "sample rod down", "retract rod in", "retract rod out", "insert rod in", "insert rod out", "wheel GV open", "wheel GV close", "vent source", "pump source", "shutdown"]
              }
            }
            n138 = shared-variable ".\\local SCA shared var lib.lvlib\\New Command?"(FALSE ("New Command?")) -> ()  [unwired: 1 in, 1 out]
          }
        }
        n139 = Index Array(array=w257, index=0) -> (element=w256:T9)
        n140 = Tick Count (ms)() -> (millisecond timer value=w255:u32)
      }
      frame "wheel GV open" {
        n141 = shared-variable "SCA-cRIO\\Mod8\\Wheel GV Actuator"(TRUE ("sc gate valve")) -> (error out=w287:errorcluster)  [unwired: 1 in]
        n142 = shared-variable ".\\local SCA shared var lib.lvlib\\Wheel GV Bypass"() -> (w290:bool)  [unwired: 1 in, 1 out]
        n143 = shared-variable "SCA-cRIO\\global SCA shared var lib.lvlib\\Wheel GV Status"(error in=w287) -> (w286:enum16{"status unclear", "closed", "open"})  [unwired: 1 out]
        n144 = Select(t=enum16{"status unclear", "closed", "open"}."open" ("x"), s=w290, f=w286) -> (s? t:f=w285:enum16{"status unclear", "closed", "open"})
        n145 = case shown="\"status unclear\", \"closed\", Default" w285 {
          tunnel: w284 -> [w297 _]
          tunnel: w279 -> [w296 w304]
          tunnel: w277 -> [w295 w303]
          tunnel: [w294 w302] -> w281
          tunnel: [w293 w301] -> w282
          tunnel: [w292 w300] -> w280
          tunnel: [w291 "wheel GV opened" ("Status Message")] -> w283
          frame "status unclear", "closed", Default {
            n146 = shared-variable ".\\local SCA shared var lib.lvlib\\Wheel GV Timeout"() -> (w298:u32)  [unwired: 1 in, 1 out]
            n147 = call "SCA state Transition Timeout Check.vi"("Start Time"=w297, "Timeout limit"=w298, "Current State In"=w295, "Modified Array of states in"=w296) -> ("Status Message"=w291:string, "millisecond timer value out"=w292:u32, "Next State"=w293:T9, "Modified Array of states out"=w294:T9[])  [unwired: 4 in]
          }
          frame "open" {
            n148 = call "Modify array of SCA states.vi"("Current State"=w303, "Array of states to process"=w304) -> ("Next State"=w301:T9, "Modified Array of states"=w302:T9[])  [unwired: 7 in]
            n149 = Tick Count (ms)() -> (millisecond timer value=w300:u32)
          }
        }
      }
      frame "wheel GV close" {
        n150 = shared-variable "SCA-cRIO\\global SCA shared var lib.lvlib\\Retract Rod Status"() -> (w323:T6)  [unwired: 1 in, 1 out]
        n151 = shared-variable "SCA-cRIO\\global SCA shared var lib.lvlib\\Insert Rod Status"() -> (w321:T6)  [unwired: 1 in, 1 out]
        n152 = shared-variable ".\\local SCA shared var lib.lvlib\\Retract Rod Bypass"() -> (w317:bool)  [unwired: 1 in, 1 out]
        n153 = shared-variable ".\\local SCA shared var lib.lvlib\\Insert Rod Bypass"() -> (w319:bool)  [unwired: 1 in, 1 out]
        n154 = Equal?(x=w321, y=Horizontal_Rod_states."rod out" ("Enum")) -> (x = y?=w320:bool)
        n155 = Equal?(x=w323, y=Horizontal_Rod_states."rod out" ("Enum")) -> (x = y?=w318:bool)
        n156 = Or(x=w319, y=w320) -> (x .or. y?=w316:bool)
        n157 = Or(x=w317, y=w318) -> (x .or. y?=w315:bool)
        n158 = Build Array(w316, w315) -> (w313:bool[])
        n159 = And Array Elements(Boolean array=w313) -> (logical AND=w314:bool)
        n160 = case shown="True" w314 {
          tunnel: w313 -> [w332 _]
          tunnel: w312 -> [w328 w347]
          tunnel: w310 -> [_ w346]
          tunnel: w311 -> [_ w345]
          tunnel: ["wheel GV interlocks not satisfied" ("Status Message") w344] -> w309
          tunnel: [w325 w343] -> w307
          tunnel: [w326 w342] -> w306
          tunnel: [w327 w341] -> w305
          frame False {
            n161 = Search 1D Array(1D array=w332, element=FALSE) -> (index of element=w330:i32)  [unwired: 1 in]
            n162 = case shown="0, Default" w330 {
              tunnel: w328 -> [w333 w340]
              tunnel: [w335 w338] -> w327
              tunnel: [w334 w337] -> w326
              frame 0, Default {
                w334 = SCA_states."insert rod out" ("SC2 state")
                n163 = Insert Into Array(array=w333, index=0, new element=w334) -> (w335:T9[])
              }
              frame 1 {
                w337 = SCA_states."retract rod out" ("SC2 state")
                n164 = Insert Into Array(array=w340, index=0, new element=w337) -> (w338:T9[])
              }
            }
            n165 = Tick Count (ms)() -> (millisecond timer value=w325:u32)
          }
          frame True {
            n166 = shared-variable "SCA-cRIO\\Mod8\\Wheel GV Actuator"(FALSE ("sc gate valve")) -> (error out=w350:errorcluster)  [unwired: 1 in]
            n167 = shared-variable ".\\local SCA shared var lib.lvlib\\Wheel GV Bypass"() -> (w353:bool)  [unwired: 1 in, 1 out]
            n168 = shared-variable "SCA-cRIO\\global SCA shared var lib.lvlib\\Wheel GV Status"(error in=w350) -> (w349:enum16{"status unclear", "closed", "open"})  [unwired: 1 out]
            n169 = Select(t=enum16{"status unclear", "closed", "open"}."closed" ("x"), s=w353, f=w349) -> (s? t:f=w348:enum16{"status unclear", "closed", "open"})
            n170 = case shown="\"status unclear\", \"open\", Default" w348 {
              tunnel: w345 -> [w360 _]
              tunnel: w347 -> [w359 w367]
              tunnel: w346 -> [w358 w366]
              tunnel: [w357 w365] -> w341
              tunnel: [w356 w364] -> w342
              tunnel: [w355 w363] -> w343
              tunnel: [w354 "wheel GV closed" ("Status Message")] -> w344
              frame "status unclear", "open", Default {
                n171 = shared-variable ".\\local SCA shared var lib.lvlib\\Wheel GV Timeout"() -> (w361:u32)  [unwired: 1 in, 1 out]
                n172 = call "SCA state Transition Timeout Check.vi"("Start Time"=w360, "Timeout limit"=w361, "Current State In"=w358, "Modified Array of states in"=w359) -> ("Status Message"=w354:string, "millisecond timer value out"=w355:u32, "Next State"=w356:T9, "Modified Array of states out"=w357:T9[])  [unwired: 4 in]
              }
              frame "closed" {
                n173 = call "Modify array of SCA states.vi"("Current State"=w366, "Array of states to process"=w367) -> ("Next State"=w364:T9, "Modified Array of states"=w365:T9[])  [unwired: 7 in]
                n174 = Tick Count (ms)() -> (millisecond timer value=w363:u32)
              }
            }
          }
        }
      }
      frame "sample rod up" {
        n175 = shared-variable "SCA-cRIO\\Mod8\\Sample Rod Actuator"(FALSE ("Sample Rod Actuator")) -> (error out=w380:errorcluster)  [unwired: 1 in]
        n176 = shared-variable ".\\local SCA shared var lib.lvlib\\Sample Rod Bypass"() -> (w377:bool)  [unwired: 1 in, 1 out]
        n177 = shared-variable "SCA-cRIO\\global SCA shared var lib.lvlib\\Sample Rod status"(error in=w380) -> (w378:T7)  [unwired: 1 out]
        n178 = Select(t=Vertical_Rod_states."rod up" ("y"), s=w377, f=w378) -> (s? t:f=w376:T7)
        n179 = case shown="\"rod up\"" w376 {
          tunnel: w375 -> [w389 w395]
          tunnel: w374 -> [w388 w394]
          tunnel: w373 -> [w387 _]
          tunnel: [w383 "sample rod up" ("Status Message")] -> w371
          tunnel: [w384 w392] -> w370
          tunnel: [w385 w391] -> w369
          tunnel: [w386 w390] -> w368
          frame "status unclear", "rod down", Default {
            n180 = shared-variable ".\\local SCA shared var lib.lvlib\\Sample Rod Timeout"() -> (w382:u32)  [unwired: 1 in, 1 out]
            n181 = call "SCA state Transition Timeout Check.vi"("Start Time"=w387, "Timeout limit"=w382, "Current State In"=w388, "Modified Array of states in"=w389) -> ("Status Message"=w383:string, "millisecond timer value out"=w384:u32, "Next State"=w385:T9, "Modified Array of states out"=w386:T9[])  [unwired: 4 in]
          }
          frame "rod up" {
            n182 = call "Modify array of SCA states.vi"("Current State"=w394, "Array of states to process"=w395) -> ("Next State"=w391:T9, "Modified Array of states"=w390:T9[])  [unwired: 7 in]
            n183 = Tick Count (ms)() -> (millisecond timer value=w392:u32)
          }
        }
      }
      frame "sample rod down" {
        n184 = shared-variable "SCA-cRIO\\global SCA shared var lib.lvlib\\Retract Rod Status"() -> (w414:T6)  [unwired: 1 in, 1 out]
        n185 = shared-variable "SCA-cRIO\\global SCA shared var lib.lvlib\\Insert Rod Status"() -> (w412:T6)  [unwired: 1 in, 1 out]
        n186 = shared-variable ".\\local SCA shared var lib.lvlib\\Retract Rod Bypass"() -> (w408:bool)  [unwired: 1 in, 1 out]
        n187 = shared-variable ".\\local SCA shared var lib.lvlib\\Insert Rod Bypass"() -> (w410:bool)  [unwired: 1 in, 1 out]
        n188 = Equal?(x=w412, y=Horizontal_Rod_states."rod out" ("Enum")) -> (x = y?=w411:bool)
        n189 = Equal?(x=w414, y=Horizontal_Rod_states."rod out" ("Enum")) -> (x = y?=w409:bool)
        n190 = Or(x=w410, y=w411) -> (x .or. y?=w407:bool)
        n191 = Or(x=w408, y=w409) -> (x .or. y?=w406:bool)
        n192 = Build Array(w407, w406) -> (w404:bool[])
        n193 = And Array Elements(Boolean array=w404) -> (logical AND=w405:bool)
        n194 = case shown="True" w405 {
          tunnel: w404 -> [w423 _]
          tunnel: w403 -> [w419 w439]
          tunnel: w402 -> [_ w438]
          tunnel: w401 -> [_ w437]
          tunnel: ["sample rod down interlocks not satisfied" ("Status Message") w436] -> w400
          tunnel: [w416 w435] -> w398
          tunnel: [w417 w434] -> w397
          tunnel: [w418 w433] -> w396
          frame False {
            n195 = Search 1D Array(1D array=w423, element=FALSE) -> (index of element=w421:i32)  [unwired: 1 in]
            n196 = case shown="0, Default" w421 {
              tunnel: w419 -> [w424 w431]
              tunnel: [w426 w429] -> w418
              tunnel: [w425 w428] -> w417
              frame 0, Default {
                w425 = SCA_states."insert rod out" ("SC2 state")
                n197 = Insert Into Array(array=w424, index=0, new element=w425) -> (w426:T9[])
              }
              frame 1 {
                w428 = SCA_states."retract rod out" ("SC2 state")
                n198 = Insert Into Array(array=w431, index=0, new element=w428) -> (w429:T9[])
              }
            }
            n199 = Tick Count (ms)() -> (millisecond timer value=w416:u32)
          }
          frame True {
            n200 = shared-variable "SCA-cRIO\\Mod8\\Sample Rod Actuator"(TRUE ("sc gate valve")) -> (error out=w442:errorcluster)  [unwired: 1 in]
            n201 = shared-variable ".\\local SCA shared var lib.lvlib\\Sample Rod Bypass"() -> (w444:bool)  [unwired: 1 in, 1 out]
            n202 = shared-variable "SCA-cRIO\\global SCA shared var lib.lvlib\\Sample Rod status"(error in=w442) -> (w441:T7)  [unwired: 1 out]
            n203 = Select(t=Vertical_Rod_states."rod up" ("y"), s=w444, f=w441) -> (s? t:f=w440:T7)
            n204 = case shown="\"status unclear\", \"rod up\", Default" w440 {
              tunnel: w437 -> [w451 _]
              tunnel: w439 -> [w450 w458]
              tunnel: w438 -> [w449 w457]
              tunnel: [w448 w456] -> w433
              tunnel: [w447 w455] -> w434
              tunnel: [w446 w454] -> w435
              tunnel: [w445 "sample rod down" ("Status Message")] -> w436
              frame "status unclear", "rod up", Default {
                n205 = shared-variable ".\\local SCA shared var lib.lvlib\\Sample Rod Timeout"() -> (w452:u32)  [unwired: 1 in, 1 out]
                n206 = call "SCA state Transition Timeout Check.vi"("Start Time"=w451, "Timeout limit"=w452, "Current State In"=w449, "Modified Array of states in"=w450) -> ("Status Message"=w445:string, "millisecond timer value out"=w446:u32, "Next State"=w447:T9, "Modified Array of states out"=w448:T9[])  [unwired: 4 in]
              }
              frame "rod down" {
                n207 = call "Modify array of SCA states.vi"("Current State"=w457, "Array of states to process"=w458) -> ("Next State"=w455:T9, "Modified Array of states"=w456:T9[])  [unwired: 7 in]
                n208 = Tick Count (ms)() -> (millisecond timer value=w454:u32)
              }
            }
          }
        }
      }
      frame "retract rod in" {
        n209 = shared-variable "SCA-cRIO\\global SCA shared var lib.lvlib\\Sample Rod status"() -> (w463:T7)  [unwired: 1 in, 1 out]
        n210 = shared-variable "SCA-cRIO\\global SCA shared var lib.lvlib\\Insert Rod Status"() -> (w481:T6)  [unwired: 1 in, 1 out]
        n211 = shared-variable "SCA-cRIO\\global SCA shared var lib.lvlib\\Wheel GV Status"() -> (w483:enum16{"status unclear", "closed", "open"})  [unwired: 1 in, 1 out]
        n212 = shared-variable ".\\local SCA shared var lib.lvlib\\Wheel GV Bypass"() -> (w477:bool)  [unwired: 1 in, 1 out]
        n213 = shared-variable ".\\local SCA shared var lib.lvlib\\Sample Rod Bypass"() -> (w461:bool)  [unwired: 1 in, 1 out]
        n214 = shared-variable ".\\local SCA shared var lib.lvlib\\Insert Rod Bypass"() -> (w479:bool)  [unwired: 1 in, 1 out]
        n215 = Equal?(x=w481, y=Horizontal_Rod_states."rod out" ("Enum")) -> (x = y?=w480:bool)
        n216 = Equal?(x=w483, y=enum16{"status unclear", "closed", "open"}."open") -> (x = y?=w478:bool)
        n217 = Equal?(x=w463, y=Vertical_Rod_states."rod up") -> (x = y?=w462:bool)
        n218 = Or(x=w479, y=w480) -> (x .or. y?=w476:bool)
        n219 = Or(x=w477, y=w478) -> (x .or. y?=w475:bool)
        n220 = Or(x=w461, y=w462) -> (x .or. y?=w460:bool)
        n221 = Build Array(w476, w475, w460) -> (w473:bool[])
        n222 = And Array Elements(Boolean array=w473) -> (logical AND=w474:bool)
        n223 = case shown="False" w474 {
          tunnel: w473 -> [w491 _]
          tunnel: w472 -> [w487 w511]
          tunnel: w471 -> [_ w510]
          tunnel: w470 -> [_ w509]
          tunnel: ["retract rod in interlocks not satisfied" ("Status Message") w508] -> w468
          tunnel: [w484 w507] -> w467
          tunnel: [w485 w506] -> w466
          tunnel: [w486 w505] -> w465
          frame False {
            n224 = Search 1D Array(1D array=w491, element=FALSE) -> (index of element=w489:i32)  [unwired: 1 in]
            n225 = case shown="0, Default" w489 {
              tunnel: w487 -> [w492 w499 w503]
              tunnel: [w494 w497 w501] -> w486
              tunnel: [w493 w496 w500] -> w485
              frame 0, Default {
                w493 = SCA_states."insert rod out" ("SC2 state")
                n226 = Insert Into Array(array=w492, index=0, new element=w493) -> (w494:T9[])
              }
              frame 1 {
                w496 = SCA_states."wheel GV open" ("SC2 state")
                n227 = Insert Into Array(array=w499, index=0, new element=w496) -> (w497:T9[])
              }
              frame 2 {
                w500 = SCA_states."sample rod up" ("SC2 state")
                n228 = Insert Into Array(array=w503, index=0, new element=w500) -> (w501:T9[])
              }
            }
            n229 = Tick Count (ms)() -> (millisecond timer value=w484:u32)
          }
          frame True {
            n230 = shared-variable "SCA-cRIO\\Mod8\\Retract Rod Actuator"(TRUE ("sc gate valve")) -> (error out=w514:errorcluster)  [unwired: 1 in]
            n231 = shared-variable ".\\local SCA shared var lib.lvlib\\Retract Rod Bypass"() -> (w516:bool)  [unwired: 1 in, 1 out]
            n232 = shared-variable "SCA-cRIO\\global SCA shared var lib.lvlib\\Retract Rod Status"(error in=w514) -> (w513:T6)  [unwired: 1 out]
            n233 = Select(t=Horizontal_Rod_states."rod in", s=w516, f=w513) -> (s? t:f=w512:T6)
            n234 = case shown="\"rod in\"" w512 {
              tunnel: w509 -> [w523 _]
              tunnel: w511 -> [w522 w530]
              tunnel: w510 -> [w521 w529]
              tunnel: [w520 w528] -> w505
              tunnel: [w519 w527] -> w506
              tunnel: [w518 w526] -> w507
              tunnel: [w517 "retract rod in" ("Status Message")] -> w508
              frame "status unclear", "rod out", Default {
                n235 = shared-variable ".\\local SCA shared var lib.lvlib\\Retract Rod Timeout"() -> (w524:u32)  [unwired: 1 in, 1 out]
                n236 = call "SCA state Transition Timeout Check.vi"("Start Time"=w523, "Timeout limit"=w524, "Current State In"=w521, "Modified Array of states in"=w522) -> ("Status Message"=w517:string, "millisecond timer value out"=w518:u32, "Next State"=w519:T9, "Modified Array of states out"=w520:T9[])  [unwired: 4 in]
              }
              frame "rod in" {
                n237 = call "Modify array of SCA states.vi"("Current State"=w529, "Array of states to process"=w530) -> ("Next State"=w527:T9, "Modified Array of states"=w528:T9[])  [unwired: 7 in]
                n238 = Tick Count (ms)() -> (millisecond timer value=w526:u32)
              }
            }
          }
        }
      }
      frame "retract rod out" {
        n239 = shared-variable "SCA-cRIO\\Mod8\\Retract Rod Actuator"(FALSE ("Sample Rod Actuator")) -> (error out=w543:errorcluster)  [unwired: 1 in]
        n240 = shared-variable ".\\local SCA shared var lib.lvlib\\Retract Rod Bypass"() -> (w542:bool)  [unwired: 1 in, 1 out]
        n241 = shared-variable "SCA-cRIO\\global SCA shared var lib.lvlib\\Retract Rod Status"(error in=w543) -> (w540:T6)  [unwired: 1 out]
        n242 = Select(t=Horizontal_Rod_states."rod out" ("Enum"), s=w542, f=w540) -> (s? t:f=w539:T6)
        n243 = case shown="\"rod out\"" w539 {
          tunnel: w538 -> [w551 w558]
          tunnel: w537 -> [w550 w557]
          tunnel: w536 -> [w549 _]
          tunnel: [w545 "retract rod out" ("Status Message")] -> w534
          tunnel: [w548 w555] -> w533
          tunnel: [w547 w554] -> w532
          tunnel: [w546 w553] -> w531
          frame "status unclear", "rod in", Default {
            n244 = shared-variable ".\\local SCA shared var lib.lvlib\\Retract Rod Timeout"() -> (w552:u32)  [unwired: 1 in, 1 out]
            n245 = call "SCA state Transition Timeout Check.vi"("Start Time"=w549, "Timeout limit"=w552, "Current State In"=w550, "Modified Array of states in"=w551) -> ("Status Message"=w545:string, "millisecond timer value out"=w548:u32, "Next State"=w547:T9, "Modified Array of states out"=w546:T9[])  [unwired: 4 in]
          }
          frame "rod out" {
            n246 = call "Modify array of SCA states.vi"("Current State"=w557, "Array of states to process"=w558) -> ("Next State"=w554:T9, "Modified Array of states"=w553:T9[])  [unwired: 7 in]
            n247 = Tick Count (ms)() -> (millisecond timer value=w555:u32)
          }
        }
      }
      frame "insert rod in" {
        n248 = shared-variable "SCA-cRIO\\global SCA shared var lib.lvlib\\Retract Rod Status"() -> (w581:T6)  [unwired: 1 in, 1 out]
        n249 = shared-variable "SCA-cRIO\\global SCA shared var lib.lvlib\\Sample Rod status"() -> (w571:T7)  [unwired: 1 in, 1 out]
        n250 = shared-variable "SCA-cRIO\\global SCA shared var lib.lvlib\\Wheel GV Status"() -> (w583:enum16{"status unclear", "closed", "open"})  [unwired: 1 in, 1 out]
        n251 = shared-variable ".\\local SCA shared var lib.lvlib\\Wheel GV Bypass"() -> (w577:bool)  [unwired: 1 in, 1 out]
        n252 = shared-variable ".\\local SCA shared var lib.lvlib\\Sample Rod Bypass"() -> (w569:bool)  [unwired: 1 in, 1 out]
        n253 = shared-variable ".\\local SCA shared var lib.lvlib\\Retract Rod Bypass"() -> (w579:bool)  [unwired: 1 in, 1 out]
        n254 = Equal?(x=w581, y=Horizontal_Rod_states."rod out" ("Enum")) -> (x = y?=w580:bool)
        n255 = Equal?(x=w583, y=enum16{"status unclear", "closed", "open"}."open") -> (x = y?=w578:bool)
        n256 = Equal?(x=w571, y=Vertical_Rod_states."rod up") -> (x = y?=w570:bool)
        n257 = Or(x=w579, y=w580) -> (x .or. y?=w576:bool)
        n258 = Or(x=w577, y=w578) -> (x .or. y?=w575:bool)
        n259 = Or(x=w569, y=w570) -> (x .or. y?=w568:bool)
        n260 = Build Array(w576, w575, w568) -> (w573:bool[])
        n261 = And Array Elements(Boolean array=w573) -> (logical AND=w574:bool)
        n262 = case shown="True" w574 {
          tunnel: w573 -> [w591 _]
          tunnel: w566 -> [w587 w611]
          tunnel: w565 -> [_ w610]
          tunnel: w564 -> [_ w609]
          tunnel: ["retract rod in interlocks not satisfied" ("Status Message") w608] -> w563
          tunnel: [w584 w607] -> w559
          tunnel: [w585 w606] -> w560
          tunnel: [w586 w605] -> w561
          frame False {
            n263 = Search 1D Array(1D array=w591, element=FALSE) -> (index of element=w589:i32)  [unwired: 1 in]
            n264 = case shown="2" w589 {
              tunnel: w587 -> [w592 w599 w603]
              tunnel: [w594 w597 w601] -> w586
              tunnel: [w593 w596 w600] -> w585
              frame 0, Default {
                w593 = SCA_states."retract rod out" ("SC2 state")
                n265 = Insert Into Array(array=w592, index=0, new element=w593) -> (w594:T9[])
              }
              frame 1 {
                w596 = SCA_states."wheel GV open" ("SC2 state")
                n266 = Insert Into Array(array=w599, index=0, new element=w596) -> (w597:T9[])
              }
              frame 2 {
                w600 = SCA_states."sample rod up" ("SC2 state")
                n267 = Insert Into Array(array=w603, index=0, new element=w600) -> (w601:T9[])
              }
            }
            n268 = Tick Count (ms)() -> (millisecond timer value=w584:u32)
          }
          frame True {
            n269 = shared-variable "SCA-cRIO\\Mod8\\Insert Rod Actuator"(TRUE ("sc gate valve")) -> (error out=w614:errorcluster)  [unwired: 1 in]
            n270 = shared-variable ".\\local SCA shared var lib.lvlib\\Insert Rod Bypass"() -> (w616:bool)  [unwired: 1 in, 1 out]
            n271 = shared-variable "SCA-cRIO\\global SCA shared var lib.lvlib\\Insert Rod Status"(error in=w614) -> (w613:T6)  [unwired: 1 out]
            n272 = Select(t=Horizontal_Rod_states."rod in", s=w616, f=w613) -> (s? t:f=w612:T6)
            n273 = case shown="\"status unclear\", \"rod out\", Default" w612 {
              tunnel: w609 -> [w623 _]
              tunnel: w611 -> [w622 w630]
              tunnel: w610 -> [w621 w629]
              tunnel: [w620 w628] -> w605
              tunnel: [w619 w627] -> w606
              tunnel: [w618 w626] -> w607
              tunnel: [w617 "insert rod in" ("Status Message")] -> w608
              frame "status unclear", "rod out", Default {
                n274 = shared-variable ".\\local SCA shared var lib.lvlib\\Insert Rod Timeout"() -> (w624:u32)  [unwired: 1 in, 1 out]
                n275 = call "SCA state Transition Timeout Check.vi"("Start Time"=w623, "Timeout limit"=w624, "Current State In"=w621, "Modified Array of states in"=w622) -> ("Status Message"=w617:string, "millisecond timer value out"=w618:u32, "Next State"=w619:T9, "Modified Array of states out"=w620:T9[])  [unwired: 4 in]
              }
              frame "rod in" {
                n276 = call "Modify array of SCA states.vi"("Current State"=w629, "Array of states to process"=w630) -> ("Next State"=w627:T9, "Modified Array of states"=w628:T9[])  [unwired: 7 in]
                n277 = Tick Count (ms)() -> (millisecond timer value=w626:u32)
              }
            }
          }
        }
      }
      frame "insert rod out" {
        n278 = shared-variable "SCA-cRIO\\Mod8\\Insert Rod Actuator"(FALSE ("Sample Rod Actuator")) -> (error out=w643:errorcluster)  [unwired: 1 in]
        n279 = shared-variable ".\\local SCA shared var lib.lvlib\\Insert Rod Bypass"() -> (w642:bool)  [unwired: 1 in, 1 out]
        n280 = shared-variable "SCA-cRIO\\global SCA shared var lib.lvlib\\Insert Rod Status"(error in=w643) -> (w631:T6)  [unwired: 1 out]
        n281 = Select(t=Horizontal_Rod_states."rod out" ("Enum"), s=w642, f=w631) -> (s? t:f=w640:T6)
        n282 = case shown="\"rod out\"" w640 {
          tunnel: w639 -> [w651 w658]
          tunnel: w638 -> [w650 w657]
          tunnel: w637 -> [w649 _]
          tunnel: [w645 "insert rod out" ("Status Message")] -> w632
          tunnel: [w648 w655] -> w635
          tunnel: [w647 w654] -> w634
          tunnel: [w646 w653] -> w633
          frame "status unclear", "rod in", Default {
            n283 = shared-variable ".\\local SCA shared var lib.lvlib\\Insert Rod Timeout"() -> (w652:u32)  [unwired: 1 in, 1 out]
            n284 = call "SCA state Transition Timeout Check.vi"("Start Time"=w649, "Timeout limit"=w652, "Current State In"=w650, "Modified Array of states in"=w651) -> ("Status Message"=w645:string, "millisecond timer value out"=w648:u32, "Next State"=w647:T9, "Modified Array of states out"=w646:T9[])  [unwired: 4 in]
          }
          frame "rod out" {
            n285 = call "Modify array of SCA states.vi"("Current State"=w657, "Array of states to process"=w658) -> ("Next State"=w654:T9, "Modified Array of states"=w653:T9[])  [unwired: 7 in]
            n286 = Tick Count (ms)() -> (millisecond timer value=w655:u32)
          }
        }
      }
      frame "change sample start" {
        n287 = call "Modify array of SCA states.vi"("Current State"=w661, "Array of states to process"=w663) -> ("Next State"=w660:T9, "Modified Array of states"=w662:T9[])  [unwired: 7 in]
        n288 = shared-variable ".\\local SCA shared var lib.lvlib\\Changing Sample"(TRUE ("Changing Sample")) -> ()  [unwired: 1 in, 1 out]
        n289 = Tick Count (ms)() -> (millisecond timer value=w664:u32)
      }
      frame "rotate wheel" {
        # "Slow down for short moves"
        # "in motor steps"
        # "The counter logic here (along with \"wait position\") doesn't appear to have a clear purpose.  Doesn't appear that the failure state could ever be acheived as the max timer"
        n290 = shared-variable ".\\local SCA shared var lib.lvlib\\Motor Status"(FALSE ("Motor Status")) -> (error out=w675:errorcluster)  [unwired: 1 in]
        n291 = shared-variable "SCA-cRIO\\global SCA shared var lib.lvlib\\New Move"() -> (w672:dbl)  [unwired: 1 in, 1 out]
        n292 = Absolute Value(x=w672) -> (abs(x)=w673:dbl)
        n293 = shared-variable ".\\local SCA shared var lib.lvlib\\Execute Move"(error in=w675) -> (w679:bool)  [unwired: 1 out]
        n294 = Less?(x=w673, y=100.0) -> (x < y?=w670:bool)
        n295 = case shown="True" w670 {
          tunnel: [w686 100.0] -> w669
          tunnel: [w686 1000.0] -> w668
          frame False {
            w686 = 10000.0
          }
          frame True {
          }
        }
        n296 = xnode "Straight-Line Move"("resource"=w685, "execute"=w679, "position"=w672, "velocity"=w669, "acceleration"=w669, "deceleration"=w669, "accel. jerk"=w668, "decel. jerk"=w668) -> ("error out"=→"Rotate Wheel error":errorcluster, "done"=w666:bool)  [unwired: 1 in, 1 out]
        "Rotation done" <- w666
        n297 = Not(x=w666) -> (.not. x?=w676:bool)
        n298 = shared-variable ".\\local SCA shared var lib.lvlib\\Execute Move"(w676) -> ()  [unwired: 1 in, 1 out]
        n299 = Select(t=SCA_states."check position" ("SC2 state"), s=w666, f=SCA_states."rotate wheel" ("SC2 state")) -> (s? t:f=w677:T9)
      }
      frame "check position" {
        n300 = Tick Count (ms)() -> (millisecond timer value=w709:u32)
        n301 = shared-variable ".\\local SCA shared var lib.lvlib\\Rotate Wheel timeout"() -> (w714:u32)  [unwired: 1 in, 1 out]
        n302 = shared-variable ".\\local SCA shared var lib.lvlib\\Rotate Wheel Minimum Time"() -> (w711:u32)  [unwired: 1 in, 1 out]
        n303 = Subtract(x=w709, y=w712) -> (x-y=w713:u32)
        n304 = Greater?(x=w714, y=w713) -> (0:w706:bool)
        n305 = Subtract(x=w709, y=w715) -> (x-y=w710:u32)
        n306 = Less?(x=w711, y=w710) -> (x < y?=w708:bool)
        n307 = And(x=w706, y=w708) -> (x .and. y?=w707:bool)
        n308 = case shown="True" w707 {
          tunnel: w723 -> [w730 w781]
          tunnel: [w726 w780] -> w722
          tunnel: [w724 w779] -> w721
          tunnel: [w729 w778] -> w720
          tunnel: w719 -> [_ w777]
          tunnel: w718 -> [w731 w776]
          tunnel: [w728 w775] -> w717
          tunnel: [w732 w774] -> w716
          tunnel: w715 -> [w725 w773]
          tunnel: w712 -> [w727 w772]
          tunnel: w706 -> [w733 _]
          frame False {
            n309 = case shown="False" w733 {
              tunnel: [w745 "waiting to check position"] -> w732
              tunnel: w731 -> [w739 w761]
              tunnel: w730 -> [w740 w762]
              tunnel: [w744 w762] -> w729
              tunnel: [w743 w761] -> w728
              tunnel: w727 -> [w736 w760]
              tunnel: [w737 w760] -> w726
              tunnel: w725 -> [w735 w759]
              tunnel: [w734 w759] -> w724
              frame False {
                # "Timeout reached"
                n310 = shared-variable ".\\local SCA shared var lib.lvlib\\Step Window Radius"() -> (w738:u8)  [unwired: 1 in, 1 out]
                n311 = Less?(x=w738, y=u8 2) -> (x < y?=w741:bool)
                n312 = case shown="False" w741 {
                  tunnel: ["Wheel rotation timed out" "relaxing precision of wheel rotation"] -> w745
                  tunnel: [SCA_states."wait" ("SC2 state") w757] -> w744
                  tunnel: [w749 w756] -> w743
                  tunnel: w740 -> [_ w757]
                  tunnel: w739 -> [_ w756]
                  tunnel: w738 -> [_ w755]
                  tunnel: [w748 w753] -> w737
                  tunnel: w736 -> [w748 _]
                  tunnel: w735 -> [w747 w752]
                  tunnel: [w747 w752] -> w734
                  frame False {
                    w749 = T9[] [enum."wait"] items=["initialize", "wait", "change sample start", "change sample", "check position", "rotate wheel", "sample change complete", "sample rod up", "sample rod down", "retract rod in", "retract rod out", "insert rod in", "insert rod out", "wheel GV open", "wheel GV close", "vent source", "pump source", "shutdown"]
                    n313 = shared-variable ".\\local SCA shared var lib.lvlib\\Motor Status"(TRUE ("Motor Status")) -> ()  [unwired: 1 in, 1 out]
                  }
                  frame True {
                    # "Add extra step to window radius"
                    n314 = Tick Count (ms)() -> (millisecond timer value=w753:u32)
                    n315 = Increment(x=w755) -> (x+1=w754:u8)
                    n316 = shared-variable ".\\local SCA shared var lib.lvlib\\Step Window Radius"(w754) -> ()  [unwired: 1 in, 1 out]
                  }
                }
              }
              frame True {
                # "Haven't met minimum wait time yet"
              }
            }
          }
          frame True {
            # "For long moves, shift \ntarget position"
            # "14-bit encoder # steps"
            # "Motor steps per revolution"
            # "Move in motor steps"
            n317 = shared-variable ".\\local SCA shared var lib.lvlib\\Step Window Radius"() -> (w771:u8)  [unwired: 1 in, 1 out]
            n318 = shared-variable "SCA-cRIO\\global SCA shared var lib.lvlib\\Encoder position"() -> (w792:i16)  [unwired: 1 in, 1 out]
            n319 = shared-variable ".\\local SCA shared var lib.lvlib\\Rollover Sample"() -> (w791:i8)  [unwired: 1 in, 1 out]
            n320 = shared-variable ".\\local SCA shared var lib.lvlib\\Encoder Offset"() -> (w793:i16)  [unwired: 1 in, 1 out]
            n321 = shared-variable ".\\local SCA shared var lib.lvlib\\New sample"() -> (w790:i8)  [unwired: 1 in, 1 out]
            n322 = call "SCA Sample-Encoder conversion.vi"("Step Window Radius"=w771, "Rollover Sample"=w791, "Encoder Offset"=w792, "Encoder Position"=w793, "Desired Sample"=w790) -> ("Window limit 1"=→"Window Limit 1":i16, "Within Range?"=w782:bool, "Encoder destination"=w794:i16, "Window limit 2"=→"Window Limit 2":i16, "New move (encoder steps)"=w787:i16)  [unwired: 2 in]
            "Encoder Destination" <- w794
            "In Range?" <- w782
            n323 = To Double Precision Float(number=w787) -> (double precision float=w783:dbl)
            n324 = Divide(x=50000.0, y=16384.0) -> (x/y=w786:dbl)
            n325 = shared-variable "SCA-cRIO\\global SCA shared var lib.lvlib\\Encoder Destination"(w794) -> ()  [unwired: 1 in, 1 out]
            n326 = shared-variable ".\\local SCA shared var lib.lvlib\\Motor Status"(w782) -> ()  [unwired: 1 in, 1 out]
            n327 = Multiply(x=w786, y=w783) -> (x*y=w795:dbl)
            n328 = Round To Nearest(number=w795) -> (nearest integer value=w765:dbl)
            n329 = Absolute Value(x=w765) -> (abs(x)=w764:dbl)
            n330 = Less?(x=w764, y=20.0) -> (x < y?=w767:bool)
            n331 = case shown="True" w782 {
              tunnel: [SCA_states."rotate wheel" ("SC2 state") w808] -> w778
              tunnel: ["rotating sample wheel" "rotation complete"] -> w774
              tunnel: [w796 w807] -> w775
              tunnel: [w797 w801] -> w779
              tunnel: [w798 w801] -> w780
              tunnel: w773 -> [_ _]
              tunnel: w772 -> [w798 _]
              tunnel: w781 -> [_ w806]
              tunnel: w776 -> [w796 w805]
              tunnel: w777 -> [_ w803]
              frame False {
                # "wheel not in correct position, rotate again"
                n332 = Tick Count (ms)() -> (millisecond timer value=w797:u32)
              }
              frame True {
                n333 = call "Modify array of SCA states.vi"("Current State"=w806, "Array of states to process"=w805) -> ("Next State"=w808:T9, "Modified Array of states"=w807:T9[])  [unwired: 7 in]
                n334 = xnode "Straight-Line Move"("resource"=w803, "execute"=FALSE) -> ()  [unwired: 8 in, 6 out]
                n335 = Tick Count (ms)() -> (millisecond timer value=w801:u32)
              }
            }
            n336 = Subtract(x=w765, y=10.0) -> (x-y=w769:dbl)
            n337 = Select(t=w765, s=w767, f=w769) -> (s? t:f=w770:dbl)
            "New Move" <- w770
            n338 = shared-variable "SCA-cRIO\\global SCA shared var lib.lvlib\\New Move"(w770) -> ()  [unwired: 1 in, 1 out]
          }
        }
      }
      frame "sample change complete" {
        n339 = call "Modify array of SCA states.vi"("Current State"=w838, "Array of states to process"=w839) -> ("Next State"=w836:T9, "Modified Array of states"=w837:T9[])  [unwired: 7 in]
        n340 = shared-variable ".\\local SCA shared var lib.lvlib\\Changing Sample"(FALSE ("Changing Sample")) -> (error out=w840:errorcluster)  [unwired: 1 in]
        n341 = Tick Count (ms)() -> (millisecond timer value=w842:u32)
        n342 = shared-variable ".\\local SCA shared var lib.lvlib\\Motor Status"(TRUE ("Motor Status"), error in=w840) -> ()  [unwired: 1 out]
      }
    }
    "action" <- w228
    "SCA next state" <- w226
    n343 = shared-variable "SCA-cRIO\\global SCA shared var lib.lvlib\\Status Message"(w231) -> ()  [unwired: 1 in, 1 out]
    n344 = call "Wait Until Next Multiple"("Count(mSec)"=u32 5) -> ()  [unwired: 1 out]
  }
  n345 = while {
    shift-right: [w850] -> _
    shift-left: timestamp(0 s since 1904-01-01) -> [w849]
    stop <- FALSE stop-if-true
    # "SCA command monitor -- when timestamp updated, new command processed"
    n346 = shared-variable "SCA-cRIO\\global SCA shared var lib.lvlib\\SM Command"() -> (w846:T4, error out=w845:errorcluster, w851:timestamp)  [unwired: 1 in]
    "SCA Command" <- w846
    n347 = Wait Until Next ms Multiple(millisecond multiple=u32 50) -> ()  [unwired: 1 out]
    n348 = Equal?(x=w851, y=w849) -> (x = y?=w852:bool)
    n349 = case shown="False" w852 {
      tunnel: w851 -> [w861 _]
      tunnel: [w861 w945] -> w850
      tunnel: w849 -> [_ w945]
      tunnel: w846 -> [w860 _]
      tunnel: w845 -> [w856 w944]
      tunnel: [w853 w944] -> w844
      frame False {
        n350 = case shown="\"Close ion source GV\"" w860 {
          tunnel: [SCA_states."wait" ("SC2 state") SCA_states."insert rod out" ("SC2 state") SCA_states."insert rod in" ("SC2 state") SCA_states."retract rod out" ("SC2 state") SCA_states."retract rod in" ("SC2 state") SCA_states."sample rod up" ("SC2 state") SCA_states."sample rod down" ("SC2 state") SCA_states."wheel GV open" ("SC2 state") SCA_states."wheel GV close" ("SC2 state") SCA_states."wait" ("SC2 state") SCA_states."wait" ("SC2 state") SCA_states."pump source" ("SC2 state") SCA_states."vent source" ("SC2 state") w892 w904 w919 w930 SCA_states."initialize" ("SC2 state")] -> w859
          tunnel: w856 -> [w863 w864 w866 w868 w870 w872 w874 w876 w878 w880 w882 w884 w886 w890 w902 w917 w929 w943]
          tunnel: [w863 w864 w866 w868 w870 w872 w874 w876 w878 w880 w882 w884 w886 w888 w900 w915 w928 w943] -> w855
          frame "Wait", Default {
          }
          frame "Retract insert rod" {
          }
          frame "Insert insert rod" {
          }
          frame "Retract retract rod" {
          }
          frame "Insert retract rod" {
          }
          frame "Retract sample rod" {
          }
          frame "Insert sample rod" {
          }
          frame "Open wheel GV" {
          }
          frame "Close wheel GV" {
          }
          frame "Open ion source GV" {
          }
          frame "Close ion source GV" {
          }
          frame "Pump out source" {
          }
          frame "Vent source" {
          }
          frame "Rotate wheel" {
            n351 = shared-variable ".\\local SCA shared var lib.lvlib\\Motor Status"(error in=w890) -> (w891:bool, error out=w889:errorcluster)
            n352 = case shown="False" w891 {
              tunnel: [SCA_states."wait" ("SC2 state") SCA_states."rotate wheel" ("SC2 state")] -> w892
              tunnel: w889 -> [w893 w897]
              tunnel: [w893 w895] -> w888
              frame False {
              }
              frame True {
                n353 = shared-variable "SCA-cRIO\\global SCA shared var lib.lvlib\\Requested Sample"(error in=w897) -> (w898:u8, error out=w896:errorcluster)
                n354 = shared-variable ".\\local SCA shared var lib.lvlib\\New sample"(w898, error in=w896) -> (error out=w895:errorcluster)
              }
            }
          }
          frame "Rotate wheel randomly" {
            n355 = shared-variable ".\\local SCA shared var lib.lvlib\\Motor Status"(error in=w902) -> (w903:bool, error out=w901:errorcluster)
            n356 = case shown="True" w903 {
              tunnel: [SCA_states."wait" ("SC2 state") SCA_states."rotate wheel" ("SC2 state")] -> w904
              tunnel: w901 -> [w905 w908]
              tunnel: [w905 w907] -> w900
              frame False {
              }
              frame True {
                n357 = Random Number (0-1)() -> (number: 0 to 1=w912:dbl)
                n358 = Multiply(x=w912, y=63.0) -> (x*y=w910:dbl)
                n359 = Round Toward +Infinity(x=w910) -> (ceil(x): smallest int >= x=w913:dbl)
                n360 = To Unsigned Byte Integer(number=w913) -> (unsigned 8bit integer=w909:u8)
                n361 = shared-variable ".\\local SCA shared var lib.lvlib\\New sample"(w909, error in=w908) -> (error out=w907:errorcluster)
              }
            }
          }
          frame "Start sample change" {
            n362 = shared-variable ".\\local SCA shared var lib.lvlib\\Motor Status"(error in=w917) -> (w918:bool, error out=w916:errorcluster)
            n363 = case shown="True" w918 {
              tunnel: [SCA_states."wait" ("SC2 state") SCA_states."change sample" ("SC2 state")] -> w919
              tunnel: w916 -> [w920 w924]
              tunnel: [w920 w922] -> w915
              frame False {
              }
              frame True {
                n364 = shared-variable "SCA-cRIO\\global SCA shared var lib.lvlib\\Requested Sample"(error in=w924) -> (w925:u8, error out=w923:errorcluster)
                n365 = shared-variable ".\\local SCA shared var lib.lvlib\\New sample"(w925, error in=w923) -> (error out=w922:errorcluster)
              }
            }
          }
          frame "Start random sample change" {
            n366 = shared-variable ".\\local SCA shared var lib.lvlib\\Motor Status"(error in=w929) -> (w931:bool, error out=w927:errorcluster)
            n367 = case shown="True" w931 {
              tunnel: [SCA_states."wait" ("SC2 state") SCA_states."change sample" ("SC2 state")] -> w930
              tunnel: [w932 w935] -> w928
              tunnel: w927 -> [w932 w934]
              frame False {
              }
              frame True {
                n368 = Random Number (0-1)() -> (number: 0 to 1=w939:dbl)
                n369 = Multiply(x=w939, y=63.0) -> (x*y=w937:dbl)
                n370 = Round Toward +Infinity(x=w937) -> (ceil(x): smallest int >= x=w940:dbl)
                n371 = To Unsigned Byte Integer(number=w940) -> (unsigned 8bit integer=w936:u8)
                n372 = shared-variable ".\\local SCA shared var lib.lvlib\\New sample"(w936, error in=w934) -> (error out=w935:errorcluster)
              }
            }
          }
          frame "Shutdown" {
          }
        }
        n373 = shared-variable ".\\local SCA shared var lib.lvlib\\SCA state control"(w859) -> (error out=w857:errorcluster)  [unwired: 1 in]
        n374 = shared-variable ".\\local SCA shared var lib.lvlib\\New Command?"(TRUE ("New Command?"), error in=w857) -> (error out=w854:errorcluster)
        n375 = Merge Errors(w854, w855) -> (w853:errorcluster)
      }
      frame True {
      }
    }
    "SCA command monitor error" <- w844
    n376 = shared-variable ".\\local SCA shared var lib.lvlib\\Command Monitor loop error"(w844) -> ()  [unwired: 1 in, 1 out]
  }
  n377 = while {
    tunnel: w15 -> [w949]
    tunnel: w21 -> [w952]
    stop <- FALSE ("stop 4") stop-if-true
    w948 = 3.0 ("Delay Time (s)")
    # "GP307 readback for both controllers on SCA - Bellows readings in and around sample rods upper position; Ion source readings are in and around source region"
    n378 = call "GP307 Read-RT.vi"("Delay Time (s)"=w948, "VISA Refnum in"=w952) -> ("error out"=w950:errorcluster, "GP307 output"=w951:T5)  [unwired: 7 in, 1 out]
    "Bellows Vac Cluster" <- w951
    n379 = call "GP307 Read-RT.vi"("Delay Time (s)"=w948, "VISA Refnum in"=w949) -> ("error out"=w946:errorcluster, "GP307 output"=w947:T5)  [unwired: 7 in, 1 out]
    "Ion Source Vac Cluster" <- w947
    n380 = shared-variable "SCA-cRIO\\global SCA shared var lib.lvlib\\Bellows Vac Cluster"(w951) -> ()  [unwired: 1 in, 1 out]
    n381 = shared-variable "SCA-cRIO\\global SCA shared var lib.lvlib\\Ion Source Vac Cluster"(w947) -> ()  [unwired: 1 in, 1 out]
    n382 = Merge Errors(w950, w946) -> (w953:errorcluster)
    "Vac Readback error" <- w953
    n383 = shared-variable ".\\local SCA shared var lib.lvlib\\Vac Readback Loop error"(w953) -> ()  [unwired: 1 in, 1 out]
    n384 = Wait Until Next ms Multiple(millisecond multiple=u32 500) -> ()  [unwired: 1 out]
  }
  n385 = while {
    tunnel: w10 -> [w961]
    stop <- FALSE ("stop 3") stop-if-true
    # "Convectron readback - GP375 Convectron uses thermocouple gauge to measure pressure on wheel chamber"
    n386 = Concatenate Strings("RD" ("write buffer 2"), "\r") -> (w968:string)
    n387 = Wait Until Next ms Multiple(millisecond multiple=u32 2000) -> ()  [unwired: 1 out]
    n388 = VISA Write(VISA resource name=w961, write buffer=w968) -> (VISA resource name out=w962:refnum<visa-resource-name>, error out=w958:errorcluster)  [unwired: 1 in, 1 out]
    n389 = property class="Instr"(reference=w962, error in=w958) -> (reference out=w963:refnum<visa-resource-name>, error out=w957:errorcluster, "Bytes at Port"=w964:u32)
    n390 = VISA Read(VISA resource name=w963, byte count=w964, error in (no error)=w957) -> (read buffer=w959:string, error out=w956:errorcluster)  [unwired: 2 out]
    "Sample Wheel Convectron" <- w959
    "Convectron readback error" <- w956
    n391 = shared-variable ".\\local SCA shared var lib.lvlib\\Convectron readback loop error"(w956) -> ()  [unwired: 1 in, 1 out]
    n392 = shared-variable "SCA-cRIO\\global SCA shared var lib.lvlib\\Sample Wheel Convectron"(w959) -> ()  [unwired: 1 in, 1 out]
  }
  n393 = node-c288() -> (w6:T12)  [unwired: 4 in]
  n394 = timed-loop {
    timing: w6 -> [_]
    timing-out: [_] -> w5
    stop <- FALSE stop-if-true
    # "Encoder readback loop"
    n395 = node-c288() -> ()  [unwired: 1 in, 1 out]
    n396 = shared-variable "SCA-cRIO\\Mod6\\DIO0"() -> (w1001:bool, error out=w984:errorcluster)  [unwired: 1 in]
    n397 = shared-variable "SCA-cRIO\\Mod6\\DIO1"(error in=w984) -> (w1000:bool, error out=w983:errorcluster)
    n398 = shared-variable "SCA-cRIO\\Mod6\\DIO2"(error in=w983) -> (w991:bool, error out=w982:errorcluster)
    n399 = shared-variable "SCA-cRIO\\Mod6\\DIO3"(error in=w982) -> (w990:bool, error out=w981:errorcluster)
    n400 = shared-variable "SCA-cRIO\\Mod6\\DIO4"(error in=w981) -> (w999:bool, error out=w980:errorcluster)
    n401 = shared-variable "SCA-cRIO\\Mod6\\DIO5"(error in=w980) -> (w998:bool, error out=w979:errorcluster)
    n402 = shared-variable "SCA-cRIO\\Mod6\\DIO6"(error in=w979) -> (w997:bool, error out=w978:errorcluster)
    n403 = shared-variable "SCA-cRIO\\Mod6\\DIO7"(error in=w978) -> (w977:bool, error out=w976:errorcluster)
    n404 = shared-variable "SCA-cRIO\\Mod6\\DIO8"(error in=w976) -> (w996:bool, error out=w975:errorcluster)
    n405 = shared-variable "SCA-cRIO\\Mod6\\DIO9"(error in=w975) -> (w989:bool, error out=w974:errorcluster)
    n406 = shared-variable "SCA-cRIO\\Mod6\\DIO10"(error in=w974) -> (w995:bool, error out=w973:errorcluster)
    n407 = shared-variable "SCA-cRIO\\Mod6\\DIO11"(error in=w973) -> (w994:bool, error out=w972:errorcluster)
    n408 = shared-variable "SCA-cRIO\\Mod6\\DIO12"(error in=w972) -> (w993:bool, error out=w971:errorcluster)
    n409 = shared-variable "SCA-cRIO\\Mod6\\DIO13"(error in=w971) -> (w992:bool, error out=w970:errorcluster)
    n410 = Bundle By Name(cluster=T15 {"MSB"=FALSE, "13th bit"=FALSE, "12th bit"=FALSE, "11th bit"=FALSE, "10th bit"=FALSE, "9th bit"=FALSE, "8th bit"=FALSE, "7th bit"=FALSE, "6th bit"=FALSE, "5th bit"=FALSE, "4th bit"=FALSE, "3rd bit"=FALSE, "2nd bit"=FALSE, "LSB"=FALSE} ("Cluster"), "MSB"=w1001, "13th bit"=w1000, "12th bit"=w991, "11th bit"=w990, "10th bit"=w999, "9th bit"=w998, "8th bit"=w997, "7th bit"=w977, "6th bit"=w996, "5th bit"=w989, "4th bit"=w995, "3rd bit"=w994, "2nd bit"=w993, "LSB"=w992) -> (w1003:T15)
    n411 = call "Encoder-Decoder.vi"("Encoder data"=w1003) -> ("Raw bits"=→"Raw bits":bool[], "Converted bits"=→"Converted bits":bool[], "Encoder position"=w988:u16)  [unwired: 8 in]
    "Encoder position" <- w988
    n412 = shared-variable "SCA-cRIO\\global SCA shared var lib.lvlib\\Encoder position"(w988, error in=w970) -> (error out=w969:errorcluster)
    "Encoder error" <- w969
    n413 = shared-variable ".\\local SCA shared var lib.lvlib\\Encoder loop error"(w969) -> ()  [unwired: 1 in, 1 out]
    n414 = node-c288() -> ()  [unwired: 1 in, 1 out]
  }
  n415 = while {
    stop <- FALSE ("stop") stop-if-true
    # "Actuator-Sensor Loop"
    n416 = Wait Until Next ms Multiple(millisecond multiple=u32 50) -> ()  [unwired: 1 out]
    n417 = shared-variable "SCA-cRIO\\Mod7\\Wheel GV OPEN sensor"() -> (w1029:bool, error out=w1015:errorcluster)  [unwired: 1 in]
    n418 = shared-variable "SCA-cRIO\\Mod7\\Wheel GV CLOSED sensor"(error in=w1015) -> (w1030:bool, error out=w1014:errorcluster)
    n419 = shared-variable "SCA-cRIO\\Mod7\\Retract Rod IN sensor"() -> (w1024:bool, error out=w1017:errorcluster)  [unwired: 1 in]
    "Retract Rod IN sensor" <- w1024
    n420 = shared-variable "SCA-cRIO\\Mod7\\Retract Rod OUT sensor"(error in=w1017) -> (w1023:bool, error out=w1011:errorcluster)
    "Retract Rod OUT sensor" <- w1023
    n421 = shared-variable "SCA-cRIO\\Mod7\\Insert Rod IN sensor"() -> (w1022:bool, error out=w1016:errorcluster)  [unwired: 1 in]
    "Insert Rod IN sensor" <- w1022
    n422 = shared-variable "SCA-cRIO\\Mod7\\Insert Rod OUT sensor"(error in=w1016) -> (w1021:bool, error out=w1013:errorcluster)
    "Insert Rod OUT sensor" <- w1021
    n423 = shared-variable "SCA-cRIO\\Mod7\\Sample Rod UP sensor"() -> (w1027:bool, error out=w1018:errorcluster)  [unwired: 1 in]
    "Sample Rod UP sensor" <- w1027
    n424 = shared-variable "SCA-cRIO\\Mod7\\Sample Rod DOWN sensor"(error in=w1018) -> (w1026:bool, error out=w1012:errorcluster)
    "Sample Rod DOWN sensor" <- w1026
    n425 = Bundle By Name(cluster=T8 {"OPEN sensor"=FALSE, "Closed sensor"=FALSE} ("Gate Valve"), "OPEN sensor"=w1029, "Closed sensor"=w1030) -> (w1032:T8)
    "Wheel GV" <- w1032
    n426 = call "Horizontal Rod Sensor-State converter.vi"("IN Sensor"=w1022, "OUT Sensor"=w1021) -> ("Status"=w1020:T6)  [unwired: 8 in]
    "Insert Rod Status" <- w1020
    n427 = call "Horizontal Rod Sensor-State converter.vi"("IN Sensor"=w1024, "OUT Sensor"=w1023) -> ("Status"=w1019:T6)  [unwired: 8 in]
    "Retract Rod Status" <- w1019
    n428 = call "Vertical Rod Sensor-State converter.vi"("UP Sensor"=w1027, "DOWN Sensor"=w1026) -> ("Status"=w1025:T7)  [unwired: 8 in]
    "Sample Rod status" <- w1025
    n429 = shared-variable "SCA-cRIO\\global SCA shared var lib.lvlib\\Retract Rod Status"(w1019, error in=w1011) -> (error out=w1008:errorcluster)
    n430 = shared-variable "SCA-cRIO\\global SCA shared var lib.lvlib\\Insert Rod Status"(w1020, error in=w1013) -> (error out=w1007:errorcluster)
    n431 = call "GV status converter.vi"("Gate Valve"=w1032) -> ("GV Status"=w1028:T16)  [unwired: 10 in]
    n432 = shared-variable "SCA-cRIO\\global SCA shared var lib.lvlib\\Sample Rod status"(w1025, error in=w1012) -> (error out=w1009:errorcluster)
    n433 = shared-variable "SCA-cRIO\\global SCA shared var lib.lvlib\\Wheel GV Status"(w1028, error in=w1014) -> (error out=w1006:errorcluster)
    n434 = Merge Errors(w1009, w1008, w1007, w1006) -> (w1010:errorcluster)
    "Sensor error" <- w1010
    n435 = shared-variable ".\\local SCA shared var lib.lvlib\\Sensor Loop error"(w1010) -> ()  [unwired: 1 in, 1 out]
  }
  n436 = node-c288(w5) -> ()  [unwired: 1 out]
